vi "Initialize.vi"() -> ()   [LabVIEW 2010]
uses:
  <vilib>/Utility/miscctls.llb/LV3DPointTypeDef.ctl
  <vilib>/picture/3D Picture Control/NI_3D Picture Control.lvlib
  <vilib>/Analysis/NI_AALBase.lvlib
panel:
  in  "MagCal":bool caption="InitializeEEPROM"
  in  "Initialize EEPROM":bool caption="InitializeEEPROM"
  in  "ESCCal":bool caption="InitializeEEPROM"
  in  "TransmitterCal":bool caption="InitializeEEPROM"
  in  "AccelCal":bool caption="InitializeEEPROM"
  in  "GyroCal":bool caption="InitializeEEPROM"
  in  "Upload Flight Software":bool caption="InitializeEEPROM"
  out "Z Axis":cluster{dbl, dbl, dbl}(slide)={0.0, 519.4805194805194, -331.16883116883116} scale=-800.0..800.0
  out "Y Axis":cluster{dbl, dbl, dbl}(slide)={0.0, 519.4805194805194, -331.16883116883116} scale=-800.0..800.0
  out "X Axis":cluster{dbl, dbl, dbl}(slide)={0.0, 519.4805194805194, -331.16883116883116} scale=-800.0..800.0
  out "AUX3":dbl
  out "AUX2":dbl
  out "AUX1":dbl
  out "Mode":dbl
  out "Pitch":dbl
  out "Roll":dbl
  out "Yaw":dbl
  out "Throttle":dbl
  out "AUX3Bar":sgl(slide) scale=1000.0..2000.0
  out "AUX2Bar":sgl(slide) scale=1000.0..2000.0
  out "AUX1Bar":sgl(slide) scale=1000.0..2000.0
  out "ModeBar":sgl(slide) scale=1000.0..2000.0
  out "Right Stick":refnum<vi>(3d-picture)
  out "PitchBar":sgl(slide) scale=1000.0..2000.0
  out "RollBar":sgl(slide) scale=1000.0..2000.0
  out "Left Stick":refnum<vi>(3d-picture)
  out "ThrottleBar":sgl(slide) scale=1000.0..2000.0
  out "YawBar":sgl(slide) scale=1000.0..2000.0
  out "LargeInstructions":string
  out "AccelGUI":refnum<vi>(3d-picture)
  out "Instruction":string
  in  "OK":bool caption="InitializeEEPROM"
  in  "Cancel":bool caption="InitializeEEPROM"
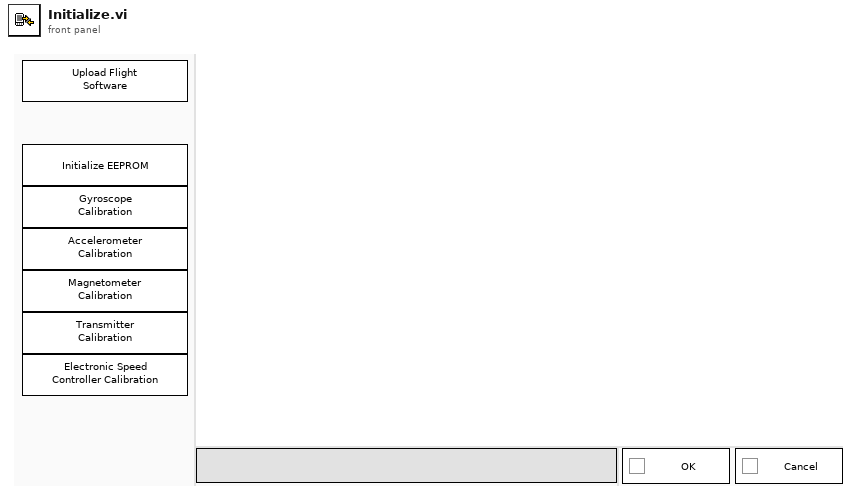
[diagram p1: front panel]
types:
  T1 = cluster{"Error":errorcluster, "GUIQueue":refnum<queue>, "TlmType":string, "Response":enum16{"Wait", "OK", "Cancel"}, "Data":dbl[][], "LeftStick":refnum<vi>, "RightStick":refnum<vi>, "XmitMax":dbl[], "XmitMin":dbl[], "NextState":string, "XmitCount":i32, "SubPanelData":string[][], "ModelRef":refnum<vi>, "Radians":dbl, "Z":sgl, "Y":sgl, "AccelIndex":i32, "AccelData":dbl[][], "AccelRaw":dbl[][], "AccelScaleFactor":dbl[], "AccelBias":dbl[], "MagMin":dbl[], "MagMax":dbl[], "IniData":string[][], "LeftStickScene":refnum<vi>, "RightStickScene":refnum<vi>, "WorkingFolder":path}
  T2 = enum8{"Enabled", "Disabled", "Disabled and Grayed Out"}
  T3 = typedef "LV3DPointTypeDef.ctl" = cluster{"X":sgl, "Y":sgl, "Z":sgl}
  T4 = cluster{"Red":sgl, "Green":sgl, "Blue":sgl, "Alpha":sgl}
  T5 = enum32{"invalid app kind", "Development System", "Run Time System", "Student Edition", "Embedded LabVIEW", "Evaluation", "Custom"}
  T6 = cluster{"State":string, "Reponse":enum16{"Wait", "OK", "Cancel"}}
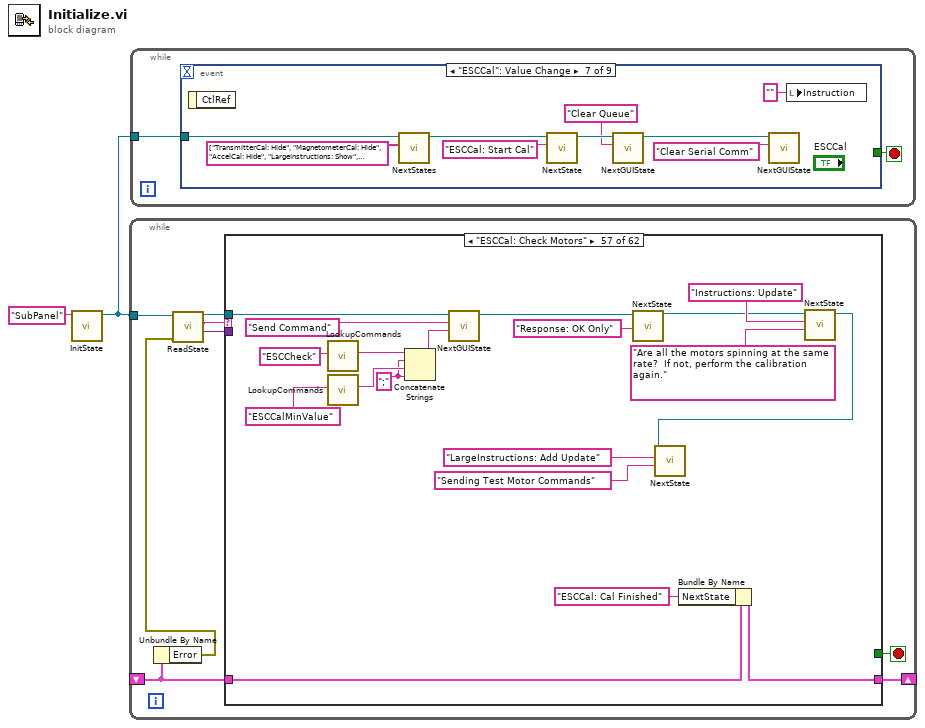
[diagram p0: block diagram]
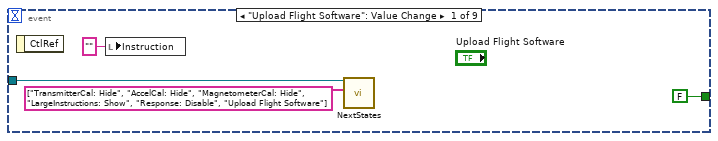
[diagram p2: hidden frame]
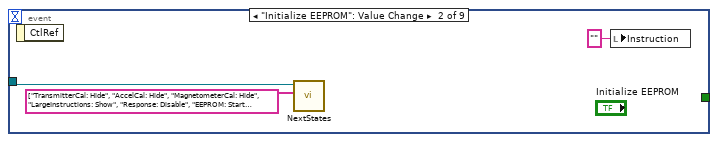
[diagram p3: hidden frame]
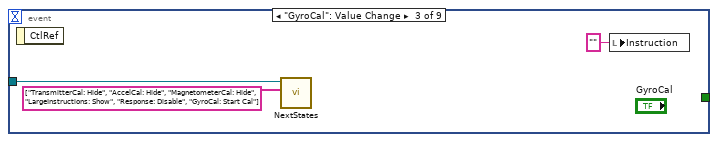
[diagram p4: hidden frame]
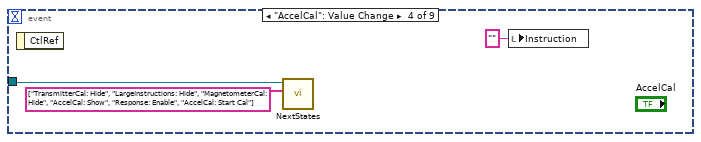
[diagram p5: hidden frame]
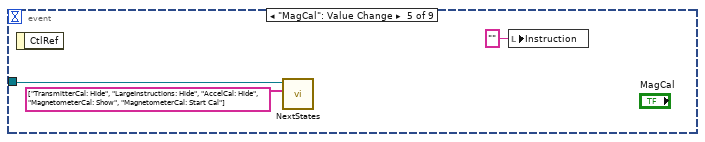
[diagram p6: hidden frame]
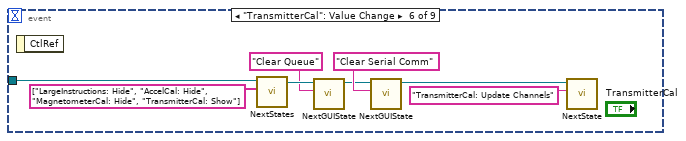
[diagram p7: hidden frame]
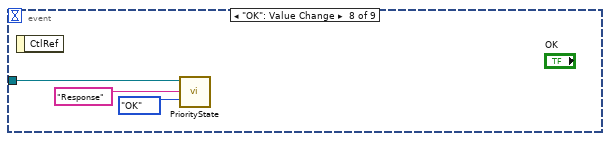
[diagram p8: hidden frame]
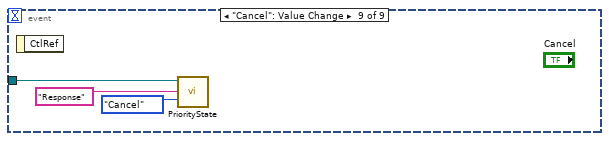
[diagram p9: hidden frame]
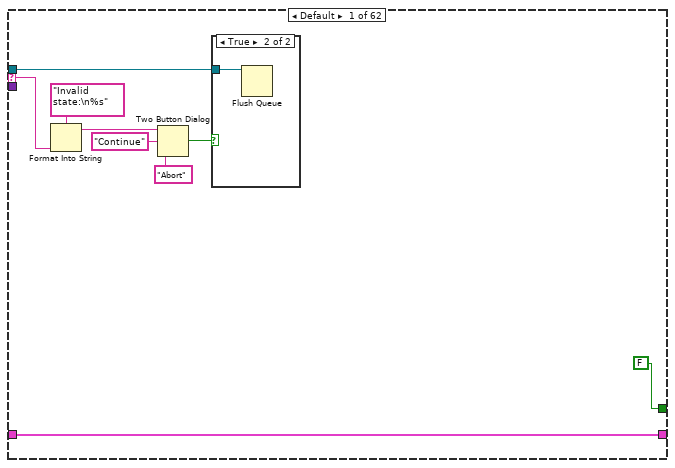
[diagram p10: hidden frame]
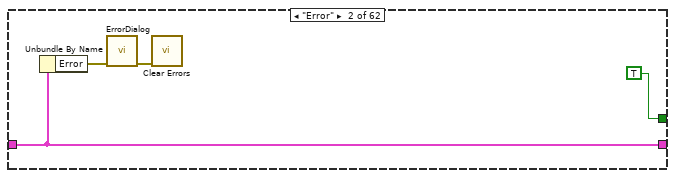
[diagram p12: hidden frame]
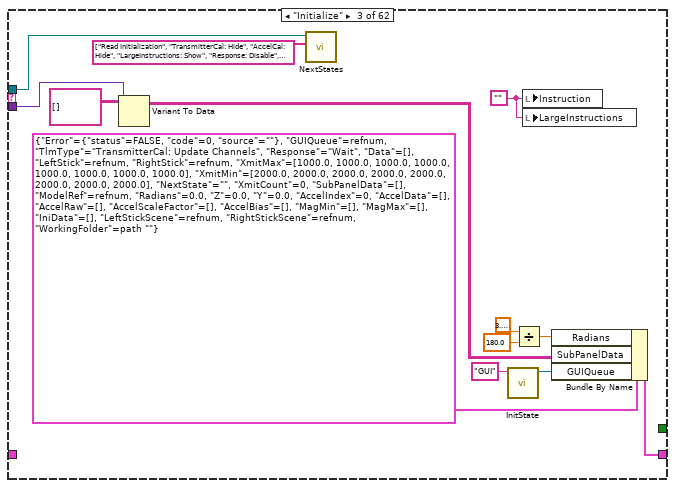
[diagram p13: hidden frame]
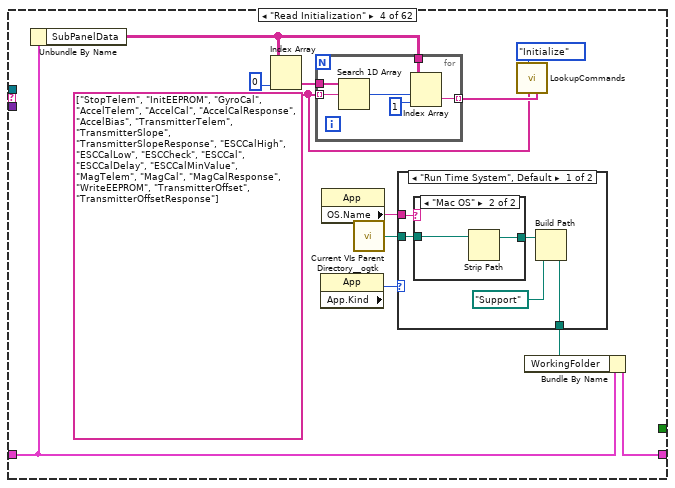
[diagram p14: hidden frame]
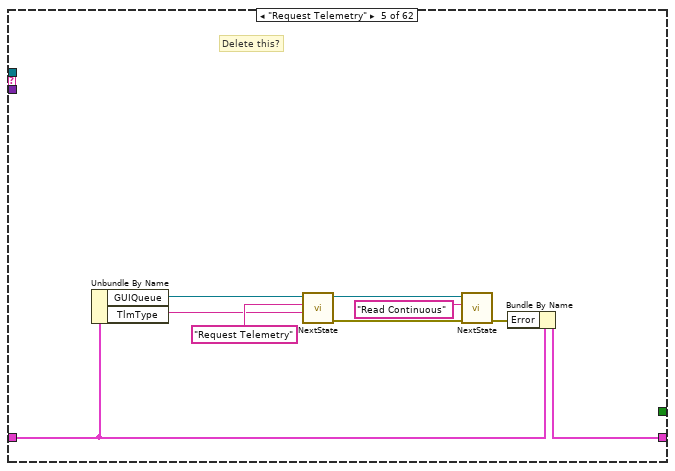
[diagram p17: hidden frame]
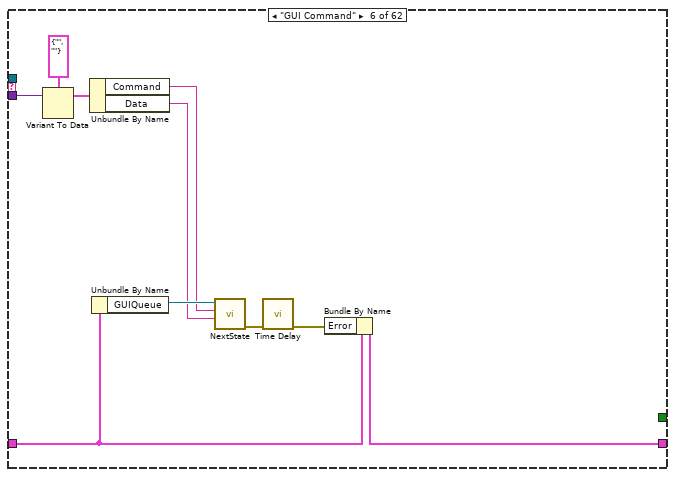
[diagram p18: hidden frame]
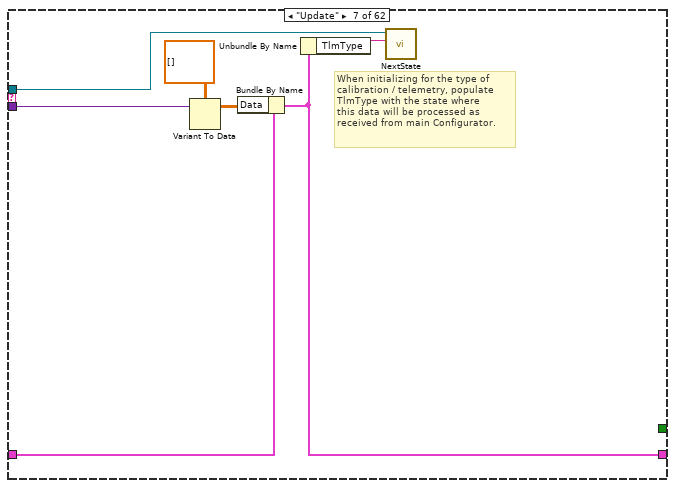
[diagram p19: hidden frame]
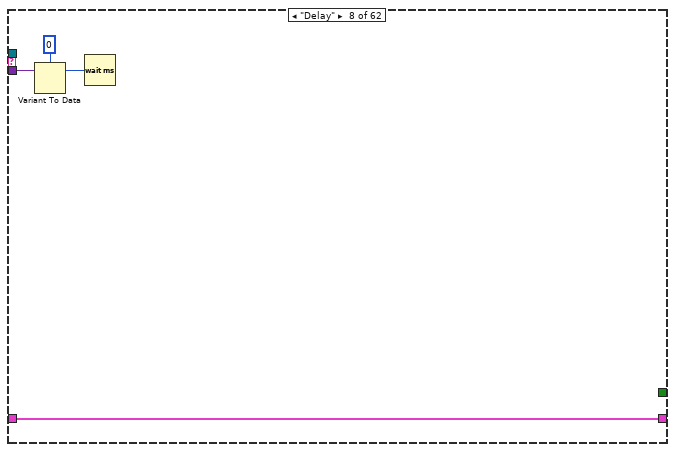
[diagram p20: hidden frame]
diagram:
  n1 = call "InitState.vi"("Name"="SubPanel" ("name (unnamed)")) -> ("Queue Out"=w1:refnum<queue>)  [unwired: 8 in, 1 out]
  n2 = while {
    tunnel: w1 -> [w7]
    shift-right: [w10] -> _
    shift-left: _ -> [w9]
    stop <- w8 stop-if-true
    n3 = Unbundle By Name(w9) -> ("Error"=w3:errorcluster)
    n4 = call "ReadState.vi"("Error In"=w3, "Queue In"=w7) -> ("Data"=w6:variant, "State"=w5:string, "Queue Out"=w4:refnum<queue>)  [unwired: 6 in, 1 out]
    n5 = case shown="\"ESCCal: Check Motors\"" w5 {
      tunnel: w4 -> [w11 _ w26 _ _ _ w86 _ w97 w104 w111 _ _ _ _ _ _ _ _ _ _ w171 w189 w217 _ w246 w266 _ w294 w323 w327 w356 w360 w389 w393 w422 w426 w458 w462 w491 _ w508 w560 w634 w650 w652 _ w695 w726 w756 w792 _ w886 w910 w944 w968 w983 w1002 _ w1030 _ w1085]
      selector: w5 -> [w17 _ _ _ _ _ _ _ _ _ _ _ _ _ _ _ _ _ _ _ w159 _ _ _ w232 _ _ _ _ _ _ _ _ _ _ _ _ _ _ _ _ _ _ _ _ _ w676 _ _ _ _ _ _ _ _ _ _ _ w1009 _ _ _]
      tunnel: w6 -> [_ _ w27 _ _ w74 w85 w94 _ _ w109 _ _ _ _ _ _ w144 w146 w155 _ _ _ _ _ _ w268 _ _ _ _ _ _ _ _ _ _ _ _ _ _ _ _ _ _ _ _ _ _ _ _ _ _ _ _ _ _ _ _ _ _ _]
      tunnel: [w16 w23 w36 w39 w70 w82 w88 w91 w95 w106 w110 w126 w130 w133 w135 w137 w138 w145 w149 w157 w162 w170 w200 w216 w233 w251 w265 w288 w304 w320 w334 w353 w367 w386 w400 w419 w433 w455 w469 w488 w495 w504 w554 w612 w648 w654 w677 w696 w719 w790 w826 w833 w882 w912 w948 w971 w989 w1006 w1008 w1021 w1041 w1082] -> w10
      tunnel: w9 -> [w16 w23 _ w40 w72 w83 w89 w91 w95 w106 w110 w126 w130 w133 w135 w137 w138 w145 w149 w157 w162 w170 w200 w216 w233 w252 w265 w288 w305 w321 w335 w354 w368 w387 w401 w420 w434 w456 w470 w489 w495 w505 w555 w613 w648 w655 w677 w697 w699 w774 w826 w834 w882 w913 w948 w971 w990 w1006 w1008 w1025 w1042 w1082]
      tunnel: [FALSE TRUE _ _ _ _ _ _ _ _ _ _ _ _ _ TRUE _ _ _ _ _ _ _ _ _ _ _ _ _ _ _ _ _ _ _ _ _ _ _ _ _ _ _ _ _ _ _ _ _ _ _ _ _ _ _ _ _ _ _ _ _ _] -> w8
      frame Default {
        n6 = Format Into String(format string="Invalid state:\n%s", w17) -> (resulting string=w18:string)  [unwired: 2 in, 1 out]
        n7 = Two Button Dialog(message=w18, 1:"Abort" ("F button name (\"Cancel\")"), 2:"Continue" ("T button name (\"OK\")")) -> (T button?=w12:bool)
        n8 = case shown="True" w12 {
          tunnel: w11 -> [_ w20]
          frame False {
          }
          frame True {
            n9 = Flush Queue(queue=w20) -> ()  [unwired: 1 in, 3 out]
          }
        }
      }
      frame "Error" {
        n10 = Unbundle By Name(w23) -> ("Error"=w22:errorcluster)
        n11 = call "ErrorDialog.vi"("error in"=w22) -> ("error out"=w21:errorcluster)  [unwired: 10 in]
        n12 = call <vilib>:"Clear Errors.vi"("error in (no error)"=w21) -> ()  [unwired: 6 in, 1 out]
      }
      frame "Initialize" {
        w32 = ""
        n13 = Variant To Data(Variant=w27, type=string[][] [] ("subarray")) -> (data=w25:string[][])  [unwired: 1 in, 1 out]
        n14 = call "NextStates.vi"("States"=string[] ["Read Initialization", "TransmitterCal: Hide", "AccelCal: Hide", "LargeInstructions: Show", "Response: Disable", "Show Welcome Message"], "Queue In"=w26) -> ()  [unwired: 8 in, 2 out]
        n15 = call "InitState.vi"("Name"="GUI") -> ("Queue Out"=w34:refnum<queue>)  [unwired: 8 in, 1 out]
        n16 = Divide(x=3.141592653589793, y=180.0) -> (x/y=w28:dbl)
        n17 = local write "Instruction"(w32) -> ()
        n18 = local write "LargeInstructions"(w32) -> ()
        n19 = Bundle By Name(cluster=T1 {"Error"={"status"=FALSE, "code"=0, "source"=""}, "GUIQueue"=refnum, "TlmType"="TransmitterCal: Update Channels", "Response"=enum."Wait", "Data"=[], "LeftStick"=refnum, "RightStick"=refnum, "XmitMax"=[1000.0, 1000.0, 1000.0, 1000.0, 1000.0, 1000.0, 1000.0, 1000.0], "XmitMin"=[2000.0, 2000.0, 2000.0, 2000.0, 2000.0, 2000.0, 2000.0, 2000.0], "NextState"="", "XmitCount"=0, "SubPanelData"=[], "ModelRef"=refnum, "Radians"=0.0, "Z"=0.0, "Y"=0.0, "AccelIndex"=0, "AccelData"=[], "AccelRaw"=[], "AccelScaleFactor"=[], "AccelBias"=[], "MagMin"=[], "MagMax"=[], "IniData"=[], "LeftStickScene"=refnum, "RightStickScene"=refnum, "WorkingFolder"=path ""}, "Radians"=w28, "SubPanelData"=w25, "GUIQueue"=w34) -> (w36:T1)
      }
      frame "Read Initialization" {
        w44 = string[] ["StopTelem", "InitEEPROM", "GyroCal", "AccelTelem", "AccelCal", "AccelCalResponse", "AccelBias", "TransmitterTelem", "TransmitterSlope", "TransmitterSlopeResponse", "ESCCalHigh", "ESCCalLow", "ESCCheck", "ESCCal", "ESCCalDelay", "ESCCalMinValue", "MagTelem", "MagCal", "MagCalResponse", "WriteEEPROM", "TransmitterOffset", "TransmitterOffsetResponse"]
        n20 = Unbundle By Name(w40) -> ("SubPanelData"=w47:string[][])
        n21 = Index Array(array=w47, index (col)=0 ("index (row)")) -> (element=w49:string[])  [unwired: 1 in]
        n22 = for {
          tunnel: w49 -> [w64]
          tunnel: w44 -> [w60] mode=indexing
          tunnel: w47 -> [w63]
          tunnel: [w59] -> w45 mode=indexing
          n23 = Search 1D Array(1D array=w64, element=w60) -> (index of element=w61:i32)  [unwired: 1 in]
          n24 = Index Array(array=w63, index (row)=w61, index (col)=1 ("disabled index (col)")) -> (element=w59:string)
        }
        n25 = property class="App"() -> ("App.Kind"=w43:T5)  [unwired: 2 in, 2 out]
        n26 = property class="App"() -> ("OS.Name"=w41:string)  [unwired: 2 in, 2 out]
        n27 = call <userlib>:"Current VIs Parent Directory__ogtk.vi"() -> ("Parent Directory (+ Relative)"=w42:path)  [unwired: 5 in]
        n28 = case shown="\"Run Time System\", Default" w43 {
          tunnel: [w54 w58] -> w38
          tunnel: w42 -> [w52 w58]
          tunnel: w41 -> [w50 _]
          frame "Run Time System", Default {
            n29 = case shown="\"Mac OS\"" w50 {
              tunnel: [w55 w57] -> w53
              tunnel: w52 -> [w55 w56]
              frame Default {
              }
              frame "Mac OS" {
                n30 = Strip Path(path=w56) -> (stripped path=w57:path)  [unwired: 1 out]
              }
            }
            n31 = Build Path(base path=w53, name or relative path=path "Support") -> (appended path=w54:path)
          }
          frame "Development System" {
          }
        }
        n32 = call "LookupCommands.vi"("CommandValues"=w45, "CommandNames"=w44, "Mode"=enum16{"Read", "Initialize"}."Initialize") -> ()  [unwired: 8 in, 1 out]
        n33 = Bundle By Name(cluster=w40, "WorkingFolder"=w38) -> (w39:T1)
      }
      frame "Request Telemetry" {
        # "Delete this?"
        n34 = Unbundle By Name(w72) -> ("GUIQueue"=w68:refnum<queue>, "TlmType"=w67:string)
        n35 = call "NextState.vi"("Data"=w67, "State"="Request Telemetry", "Queue In"=w68) -> ("Error Out"=w65:errorcluster, "Queue Out"=w66:refnum<queue>)  [unwired: 7 in]
        n36 = call "NextState.vi"("Error In"=w65, "State"="Read Continuous", "Queue In"=w66) -> ("Error Out"=w71:errorcluster)  [unwired: 7 in, 1 out]
        n37 = Bundle By Name(cluster=w72, "Error"=w71) -> (w70:T1)
      }
      frame "GUI Command" {
        n38 = Variant To Data(Variant=w74, type=cluster{"Command":string, "Data":string} {"Command"="", "Data"=""}) -> (data=w79:cluster{"Command":string, "Data":string})  [unwired: 1 in, 1 out]
        n39 = Unbundle By Name(w79) -> ("Command"=w76:string, "Data"=w75:string)
        n40 = Unbundle By Name(w83) -> ("GUIQueue"=w81:refnum<queue>)
        n41 = call "NextState.vi"("Data"=w75, "State"=w76, "Queue In"=w81) -> ("Error Out"=w78:errorcluster)  [unwired: 7 in, 1 out]
        n42 = call "Time Delay"("error in (no error)"=w78) -> ("error out"=w77:errorcluster)  [unwired: 10 in]
        n43 = Bundle By Name(cluster=w83, "Error"=w77) -> (w82:T1)
      }
      frame "Update" {
        # "When initializing for the type of\ncalibration / telemetry, populate\nTlmType with the state where\nthis data will be processed as\nreceived from main Configurator."
        n44 = Variant To Data(Variant=w85, type=dbl[][] []) -> (data=w84:dbl[][])  [unwired: 1 in, 1 out]
        n45 = Bundle By Name(cluster=w89, "Data"=w84) -> (w88:T1)
        n46 = Unbundle By Name(w88) -> ("TlmType"=w87:string)
        n47 = call "NextState.vi"("State"=w87, "Queue In"=w86) -> ()  [unwired: 8 in, 2 out]
      }
      frame "Delay" {
        n48 = Variant To Data(Variant=w94, type=u32 0 ("milliseconds to wait")) -> (data=w92:u32)  [unwired: 1 in, 1 out]
        n49 = Wait (ms)(milliseconds to wait=w92) -> ()  [unwired: 1 out]
      }
      frame "Wait For User" {
        n50 = Unbundle By Name(w95) -> ("Response"=w96:enum16{"Wait", "OK", "Cancel"})
        n51 = case shown="\"Wait\"" w96 {
          tunnel: w97 -> [_ w102]
          frame Default {
          }
          frame "Wait" {
            n52 = Bundle("State"="Wait For User", "Reponse"=enum16{"Wait", "OK", "Cancel"}."Wait") -> (w98:T6)  [unwired: 1 in]
            n53 = Enqueue Element At Opposite End(queue=w102, element=w98) -> ()  [unwired: 2 in, 3 out]
            n54 = Wait (ms)(milliseconds to wait=u32 100) -> ()  [unwired: 1 out]
          }
        }
      }
      frame "Show Welcome Message" {
        n55 = call "NextState.vi"("Data"="Welcome to the AeroQuad Configurator!\n\nThis tool is used to configure, calibrate and test your AeroQuad in preparation for flight.  Before using the Configurator, please install the Arduino IDE 1.0 or greater (found at www.arduino.cc) and install the proper drivers for your Arduino board to connect to your computer.\n\nTo setup your AeroQuad click on each of the buttons in the Initial Setup screen:\n - Upload Flight Software (advanced users can also upload directly from the Arduino IDE)\n - Initialize EEPROM (returns user configurable values to their default values)\n - Gyroscope Calibration\n - Accelerometer Calibration\n - Magnetometer Calibration (only valid with hardware configurations supporting this)\n - Transmitter Calibration\n - Electronic Speed Controller Calibration (perform this calibration with no propellers attached)\n\nAfter your AeroQuad has been properly setup, you can revisit the Initial Setup screen periodically to update  your AeroQuad configuration and calibrations as necessary.\n\nTo arm the AeroQuad motors, move the left transmitter stick to the lower right hand corner.  To disarm the motors, move the left transmitter stick to the lower left hand corner.  To perform a quick gyro/accel calibration move the left transmitter stick to the lower left hand corner and move the right transmitter stick to the lower right hand corner.\n\nFor additional help please visit www.AeroQuad.com to access our wiki documentation, help forums, and IRC chat.  Please practice safe flying, as multicopters can be dangerous if not flown with common sense.  Do as much testing as possible with the propellers not attached and only fly in approved R/C locations." ("State"), "State"="LargeInstructions: Update", "Queue In"=w104) -> ()  [unwired: 7 in, 2 out]
      }
      frame "Response" {
        w115 = enum16{"Wait", "OK", "Cancel"}."OK"  # Reponse
        # "To use the front panel OK and Cancel buttons:\nSet \"Next State\" to the state that needs to run right after the buttons are pressed.\nGo to the Reponse: Enable state to enable the buttons\nGo to Instructions: Update and send a message to tell user what happens when\n  buttons are pressed\nButtons wil automatically be disabled once either OK or Canel is pressed"
        n56 = Unbundle By Name(w110) -> ("NextState"=w112:string)
        n57 = Variant To Data(Variant=w109, type=w115) -> (data=w114:enum16{"Wait", "OK", "Cancel"})  [unwired: 1 in, 1 out]
        n58 = Equal?(x=w114, y=w115) -> (x = y?=w113:bool)
        n59 = case shown="True" w113 {
          tunnel: w112 -> [_ w121]
          tunnel: w111 -> [w119 w122]
          tunnel: [w116 w120] -> w108
          frame False {
            n60 = call "NextState.vi"("Data"="Operation cancelled." ("State"), "State"="Instructions: Update", "Queue In"=w119) -> ("Queue Out"=w116:refnum<queue>)  [unwired: 7 in, 1 out]
          }
          frame True {
            n61 = call "NextState.vi"("State"=w121, "Queue In"=w122) -> ("Queue Out"=w120:refnum<queue>)  [unwired: 8 in, 1 out]
          }
        }
        n62 = call "NextState.vi"("State"="Response: Disable", "Queue In"=w108) -> ()  [unwired: 8 in, 2 out]
      }
      frame "Response: Enable" {
        n63 = local write "Instruction"("" ("Instruction")) -> ()
        n64 = property on="Cancel" class="Bool"("DisabledEnum"=T2."Enabled" ("Disabled")) -> ()  [unwired: 2 in, 2 out]
        n65 = property on="OK" class="Bool"("DisabledEnum"=T2."Enabled" ("Disabled")) -> ()  [unwired: 2 in, 2 out]
      }
      frame "Response: OK Only" {
        n66 = local write "Instruction"("" ("Instruction")) -> ()
        n67 = property on="Cancel" class="Bool"("DisabledEnum"=T2."Disabled and Grayed Out" ("Disabled")) -> ()  [unwired: 2 in, 2 out]
        n68 = property on="OK" class="Bool"("DisabledEnum"=T2."Enabled" ("Disabled")) -> ()  [unwired: 2 in, 2 out]
      }
      frame "Response: Disable" {
        n69 = property on="Cancel" class="Bool"("DisabledEnum"=T2."Disabled and Grayed Out" ("Disabled")) -> ()  [unwired: 2 in, 2 out]
        n70 = property on="OK" class="Bool"("DisabledEnum"=T2."Disabled and Grayed Out" ("Disabled")) -> ()  [unwired: 2 in, 2 out]
      }
      frame "Temporary" {
        n71 = One Button Dialog(message="This feature under contruction.") -> ()  [unwired: 1 in, 1 out]
      }
      frame "Shutdown" {
      }
      frame "----------" {
      }
      frame "Instructions: Update" {
        w141 = "" ("Instruction")
        n72 = Variant To Data(Variant=w144, type=w141) -> (data=w139:string)  [unwired: 1 in, 1 out]
        n73 = Equal?(x=w139, y="Calibration... 0 %") -> (x = y?=w142:bool)
        n74 = Select(t=w141, s=w142, f=w139) -> (s? t:f=→"Instruction":string)
      }
      frame "LargeInstructions: Update" {
        n75 = Variant To Data(Variant=w146, type="" ("Instruction")) -> (data=→"LargeInstructions":string)  [unwired: 1 in, 1 out]
      }
      frame "LargeInstructions: Add Update" {
        n76 = Variant To Data(Variant=w155, type="" ("Instruction")) -> (data=w154:string)  [unwired: 1 in, 1 out]
        n77 = local read "LargeInstructions"() -> (w153:string)
        n78 = Concatenate Strings(w153, "\n\n**********\n\n" ("string"), w154) -> (w151:string)
        n79 = property on="LargeInstructions" class="Str"("Value"=w151, "Text.Scroll Position"=u32 1024) -> ()  [unwired: 2 in, 2 out]
      }
      frame "LargeInstructions: Hide", "LargeInstructions: Show" {
        n80 = Match Pattern(string=w159, regular expression="Show") -> (offset past match=w161:i32)  [unwired: 1 in, 3 out]
        n81 = Greater Or Equal To 0?(x=w161) -> (x >= 0?=w158:bool)
        n82 = property on="LargeInstructions" class="Str"("Visible"=w158) -> ()  [unwired: 2 in, 2 out]
      }
      frame "Upload Flight Software" {
        n83 = call "NextGUIState.vi"("GUI State"="Disconnect" ("State"), "Queue In"=w171) -> ("Queue Out"=w166:refnum<queue>)  [unwired: 8 in, 1 out]
        n84 = flat-sequence {
          tunnel: w166 -> [w176]
          tunnel: [w176] -> w169
          tunnel: [w175] -> w168
          tunnel: [w177] -> w164
          tunnel: [w182] -> w165
          tunnel: w169 -> [w182]
          tunnel: w168 -> [w177]
          tunnel: [w178] -> w163
          frame #0 {
            n85 = call "AeroQuadUploader.vi"() -> ("Com Port Out"=w175:refnum<visa-resource-name>)  [unwired: 11 in]
          }
          frame #1 {
            n86 = call "TestUsbSerialPort.vi"("Serial Port To Test"=w177) -> ()  [unwired: 9 in, 2 out]
            n87 = Two Button Dialog(message="Would you like to auto-connect to the AeroQuad?", 1:"No", 2:"Yes") -> (T button?=w178:bool)
          }
        }
        n88 = case shown="True" w163 {
          tunnel: w165 -> [_ w174]
          tunnel: w164 -> [_ w172]
          frame False {
          }
          frame True {
            n89 = call "NextGUIState.vi"("State Argument"=w172, "GUI State"="Remote Open Port" ("State Argument"), "Queue In"=w174) -> ()  [unwired: 7 in, 2 out]
          }
        }
      }
      frame "EEPROM: Start Initialization" {
        n90 = call "NextGUIState.vi"("GUI State"="Lock User Controls" ("State"), "Queue In"=w189) -> ("Queue Out"=w190:refnum<queue>)  [unwired: 8 in, 1 out]
        n91 = call "NextGUIState.vi"("State Argument"="Please wait, updating EEPROM..." ("State"), "GUI State"="Status" ("State"), "Queue In"=w190) -> ("Queue Out"=w211:refnum<queue>)  [unwired: 7 in, 1 out]
        n92 = call "NextGUIState.vi"("GUI State"="Clear Queue", "Queue In"=w211) -> ("Queue Out"=w208:refnum<queue>)  [unwired: 8 in, 1 out]
        n93 = call "LookupCommands.vi"("CommandName"="InitEEPROM") -> ("CommandValue"=w198:string)  [unwired: 10 in]
        n94 = call "NextGUIState.vi"("GUI State"="Clear Serial Comm", "Queue In"=w208) -> ("Queue Out"=w206:refnum<queue>)  [unwired: 8 in, 1 out]
        n95 = call "NextGUIState.vi"("State Argument"=w198, "GUI State"="Send Command" ("State"), "Queue In"=w206) -> ("Queue Out"=w212:refnum<queue>)  [unwired: 7 in, 1 out]
        n96 = call "NextGUIState.vi"("State Argument"="1000", "GUI State"="Delay String", "Queue In"=w212) -> ("Queue Out"=w193:refnum<queue>)  [unwired: 7 in, 1 out]
        n97 = call "NextGUIState.vi"("GUI State"="Update Parameters" ("State"), "Queue In"=w193) -> ("Queue Out"=w187:refnum<queue>)  [unwired: 8 in, 1 out]
        n98 = call "LookupCommands.vi"("CommandName"="WriteEEPROM") -> ("CommandValue"=w196:string)  [unwired: 10 in]
        n99 = call "NextGUIState.vi"("State Argument"=w196, "GUI State"="Send Command" ("State"), "Queue In"=w187) -> ("Queue Out"=w186:refnum<queue>)  [unwired: 7 in, 1 out]
        n100 = call "NextGUIState.vi"("State Argument"="1000", "GUI State"="Delay String", "Queue In"=w186) -> ("Queue Out"=w185:refnum<queue>)  [unwired: 7 in, 1 out]
        n101 = call "NextGUIState.vi"("State Argument"="EEPROM Initialized" ("State"), "GUI State"="Status" ("State"), "Queue In"=w185) -> ("Queue Out"=w183:refnum<queue>)  [unwired: 7 in, 1 out]
        n102 = call "NextGUIState.vi"("GUI State"="Unlock User Controls" ("State"), "Queue In"=w183) -> ()  [unwired: 8 in, 2 out]
      }
      frame "GyroCal: Start Cal" {
        n103 = call "NextGUIState.vi"("GUI State"="Clear Queue", "Queue In"=w217) -> ("Queue Out"=w227:refnum<queue>)  [unwired: 8 in, 1 out]
        n104 = call "NextGUIState.vi"("GUI State"="Clear Serial Comm", "Queue In"=w227) -> ("Queue Out"=w224:refnum<queue>)  [unwired: 8 in, 1 out]
        n105 = call "LookupCommands.vi"("CommandName"="GyroCal") -> ("CommandValue"=w214:string)  [unwired: 10 in]
        n106 = call "NextGUIState.vi"("State Argument"="Starting Gyroscope Calibration" ("State"), "GUI State"="Status" ("State"), "Queue In"=w224) -> ("Queue Out"=w225:refnum<queue>)  [unwired: 7 in, 1 out]
        n107 = call "NextGUIState.vi"("State Argument"=w214, "GUI State"="Send Command", "Queue In"=w225) -> ("Queue Out"=w218:refnum<queue>)  [unwired: 7 in, 1 out]
        n108 = call "NextGUIState.vi"("State Argument"="Gyroscope calibration complete" ("State"), "GUI State"="Status" ("State"), "Queue In"=w218) -> ()  [unwired: 7 in, 2 out]
      }
      frame "AccelCal: Hide", "AccelCal: Show" {
        n109 = Match Pattern(string=w232, regular expression="Show") -> (offset past match=w230:i32)  [unwired: 1 in, 3 out]
        n110 = Greater Or Equal To 0?(x=w230) -> (x >= 0?=w229:bool)
        n111 = property on="AccelGUI" class="SceneGraphDisp (strict)"("Visible"=w229) -> ()  [unwired: 2 in, 2 out]
      }
      frame "AccelCal: Start Cal" {
        w238 = dbl[][] [] ("AccelData")
        n112 = Unbundle By Name(w252) -> ("WorkingFolder"=w237:path, "SubPanelData"=w254:string[][])
        n113 = Index Array(array=w254, index (col)=0 ("index (row)")) -> (element=w255:string[])  [unwired: 1 in]
        n114 = Search 1D Array(1D array=w255, element="Filename") -> (index of element=w258:i32)  [unwired: 1 in]
        n115 = call "NextState.vi"("State"="AccelCal: Update Camera", "Queue In"=w246) -> ("Queue Out"=w247:refnum<queue>)  [unwired: 8 in, 1 out]
        n116 = Index Array(array=w254, index (row)=w258, index (col)=1 ("index (row)")) -> (element=w250:string)
        n117 = Build Path(base path=w237, name or relative path=w250) -> (appended path=w241:path)
        n118 = call <vilib>:"Create Object.vi"() -> ("Scene:New Object"=w262:refnum<vi>)  [unwired: 2 in, 9 out]
        n119 = call <vilib>:"Load STL Geometry.vi"("Model File"=w241) -> ("error out"=w261:errorcluster, "New Mesh Refnum"=w263:refnum<vi>)  [unwired: 9 in]
        n120 = invoke class="SceneObject" method="Set Drawable"(reference=w262, error in=w261, "Drawable"=w263) -> (reference out=w259:refnum<vi>, error out=w260:errorcluster)  [unwired: 1 in, 2 out]
        n121 = call "NextState.vi"("State"="AccelCal: Display Right Side Up", "Queue In"=w247) -> ("Queue Out"=w239:refnum<queue>)  [unwired: 8 in, 1 out]
        n122 = Bundle By Name(cluster=w252, "AccelIndex"=0, "AccelData"=w238, "AccelRaw"=w238, "Y"=sgl -38.0, "Z"=sgl 15.0, "TlmType"="AccelCal: Update", "ModelRef"=w259, "Error"=w260) -> (w251:T1)
        n123 = call "NextState.vi"("State"="AccelCal: Update Display", "Queue In"=w239) -> ("Queue Out"=w234:refnum<queue>)  [unwired: 8 in, 1 out]
        n124 = call "NextGUIState.vi"("State Argument"="Performing Accelerometer Calibration" ("State"), "GUI State"="Status" ("State"), "Queue In"=w234) -> ()  [unwired: 7 in, 2 out]
      }
      frame "AccelCal: Request Telemetry" {
        # "This will automatically go\nto AccelCal: Update\nto store data"
        n125 = Variant To Data(Variant=w268, type=FALSE) -> (data=w264:bool)  [unwired: 1 in, 1 out]
        n126 = case shown="True" w264 {
          tunnel: w266 -> [w274 w285]
          frame False {
            n127 = call "NextGUIState.vi"("GUI State"="Clear Queue" ("State"), "Queue In"=w274) -> ("Queue Out"=w276:refnum<queue>)  [unwired: 8 in, 1 out]
            n128 = call "NextGUIState.vi"("GUI State"="Clear Serial Comm" ("State"), "Queue In"=w276) -> ("Queue Out"=w272:refnum<queue>)  [unwired: 8 in, 1 out]
            n129 = local write "Instruction"("" ("Instruction")) -> ()
            n130 = call "LookupCommands.vi"("CommandName"="StopTelem") -> ("CommandValue"=w269:string)  [unwired: 10 in]
            n131 = call "NextGUIState.vi"("State Argument"=w269, "GUI State"="Request Telemetry" ("State"), "Queue In"=w272) -> ()  [unwired: 7 in, 2 out]
          }
          frame True {
            n132 = call "LookupCommands.vi"("CommandName"="AccelTelem") -> ("CommandValue"=w278:string)  [unwired: 10 in]
            n133 = call "NextGUIState.vi"("State Argument"=w278, "GUI State"="Request Telemetry" ("State"), "Queue In"=w285) -> ("Queue Out"=w283:refnum<queue>)  [unwired: 7 in, 1 out]
            n134 = call "NextGUIState.vi"("GUI State"="Read Continuous", "Queue In"=w283) -> ("Queue Out"=w280:refnum<queue>)  [unwired: 8 in, 1 out]
            n135 = call "NextState.vi"("State"="Response: Disable", "Queue In"=w280) -> ()  [unwired: 8 in, 2 out]
          }
        }
      }
      frame "AccelCal: Update Camera" {
        w290 = T3 {"X"=0.0, "Y"=0.0, "Z"=0.0} ("Target")
        n136 = Unbundle By Name(w288) -> ("Y"=w287:sgl, "Z"=w286:sgl)
        n137 = Bundle By Name(cluster=w290, "Y"=w287, "Z"=w286) -> (w289:T3)
        n138 = invoke on="AccelGUI" class="SceneGraphDisp (strict)" method="Setup Camera"("Camera Position"=w289, "Target"=w290, "Up Direction"=T3 {"X"=0.0, "Y"=1.0, "Z"=1.0} ("Target")) -> ()  [unwired: 3 in, 6 out]
      }
      frame "AccelCal: Display Right Side Up" {
        n139 = Unbundle By Name(w305) -> ("Radians"=w311:dbl, "ModelRef"=w317:refnum<vi>)
        n140 = call <vilib>:"Clear Transformation.vi"("Object Refnum In"=w317) -> ("Object Refnum Out"=w310:refnum<vi>)  [unwired: 9 in, 1 out]
        n141 = Compound Arithmetic op=MULTIPLY(0.0 ("value"), w311) -> (w313:dbl)
        n142 = call "NextState.vi"("State"="AccelCal: Update Camera", "Queue In"=w294) -> ("Queue Out"=w293:refnum<queue>)  [unwired: 8 in, 1 out]
        n143 = call <vilib>:"Rotate Object.vi"("Angle"=w313, "Axis"=cluster{"X":sgl, "Y":sgl, "Z":sgl} {"X"=0.0, "Y"=1.0, "Z"=0.0}, "Scene.Object In"=w310) -> ("Scene.Object Out"=w314:refnum<vi>)  [unwired: 7 in, 1 out]
        n144 = Compound Arithmetic op=MULTIPLY(0.0 ("value"), w311) -> (w312:dbl)
        n145 = call <vilib>:"Rotate Object.vi"("Angle"=w312, "Axis"=cluster{"X":sgl, "Y":sgl, "Z":sgl} {"X"=1.0, "Y"=0.0, "Z"=0.0}, "Scene.Object In"=w314) -> ("Scene.Object Out"=w309:refnum<vi>)  [unwired: 7 in, 1 out]
        n146 = Compound Arithmetic op=MULTIPLY(0.0 ("value"), w311) -> (w307:dbl)
        n147 = call <vilib>:"Rotate Object.vi"("Angle"=w307, "Axis"=cluster{"X":sgl, "Y":sgl, "Z":sgl} {"X"=0.0, "Y"=0.0, "Z"=1.0}, "Scene.Object In"=w309) -> ("Scene.Object Out"=w306:refnum<vi>)  [unwired: 7 in, 1 out]
        n148 = call "NextState.vi"("State"="Response: Enable", "Queue In"=w293) -> ("Queue Out"=w295:refnum<queue>)  [unwired: 8 in, 1 out]
        n149 = Bundle By Name(cluster=w305, "Z"=sgl 0.0, "NextState"="AccelCal: Wait Right Side Up", "ModelRef"=w306) -> (w304:T1)
        n150 = call "NextState.vi"("Data"="Place the AeroQuad motionless on a flat surface." ("State"), "State"="Instructions: Update", "Queue In"=w295) -> ()  [unwired: 7 in, 2 out]
      }
      frame "AccelCal: Wait Right Side Up" {
        n151 = call "NextState.vi"("Data"=TRUE, "State"="AccelCal: Request Telemetry", "Queue In"=w323) -> ()  [unwired: 7 in, 2 out]
        n152 = Bundle By Name(cluster=w321, "AccelRaw"=dbl[][] [] ("AccelData"), "AccelIndex"=0, "NextState"="AccelCal: Display Upside Down") -> (w320:T1)
      }
      frame "AccelCal: Display Upside Down" {
        n153 = Unbundle By Name(w335) -> ("Radians"=w344:dbl, "ModelRef"=w350:refnum<vi>)
        n154 = call <vilib>:"Clear Transformation.vi"("Object Refnum In"=w350) -> ("Object Refnum Out"=w343:refnum<vi>)  [unwired: 9 in, 1 out]
        n155 = call "NextState.vi"("State"="Response: Enable", "Queue In"=w327) -> ("Queue Out"=w329:refnum<queue>)  [unwired: 8 in, 1 out]
        n156 = Compound Arithmetic op=MULTIPLY(180.0 ("value"), w344) -> (w346:dbl)
        n157 = call <vilib>:"Rotate Object.vi"("Angle"=w346, "Axis"=cluster{"X":sgl, "Y":sgl, "Z":sgl} {"X"=0.0, "Y"=1.0, "Z"=0.0}, "Scene.Object In"=w343) -> ("Scene.Object Out"=w347:refnum<vi>)  [unwired: 7 in, 1 out]
        n158 = Compound Arithmetic op=MULTIPLY(0.0 ("value"), w344) -> (w345:dbl)
        n159 = call <vilib>:"Rotate Object.vi"("Angle"=w345, "Axis"=cluster{"X":sgl, "Y":sgl, "Z":sgl} {"X"=1.0, "Y"=0.0, "Z"=0.0}, "Scene.Object In"=w347) -> ("Scene.Object Out"=w342:refnum<vi>)  [unwired: 7 in, 1 out]
        n160 = Compound Arithmetic op=MULTIPLY(0.0 ("value"), w344) -> (w340:dbl)
        n161 = call "NextState.vi"("Data"="Place the AeroQuad upside down." ("State"), "State"="Instructions: Update", "Queue In"=w329) -> ("Queue Out"=w326:refnum<queue>)  [unwired: 7 in, 1 out]
        n162 = call <vilib>:"Rotate Object.vi"("Angle"=w340, "Axis"=cluster{"X":sgl, "Y":sgl, "Z":sgl} {"X"=0.0, "Y"=0.0, "Z"=1.0}, "Scene.Object In"=w342) -> ("Scene.Object Out"=w339:refnum<vi>)  [unwired: 7 in, 1 out]
        n163 = Bundle By Name(cluster=w335, "NextState"="AccelCal: Wait Upside Side Down", "ModelRef"=w339) -> (w334:T1)
        n164 = call "NextState.vi"("State"="AccelCal: Update Display", "Queue In"=w326) -> ()  [unwired: 8 in, 2 out]
      }
      frame "AccelCal: Wait Upside Side Down" {
        n165 = call "NextState.vi"("Data"=TRUE, "State"="AccelCal: Request Telemetry", "Queue In"=w356) -> ()  [unwired: 7 in, 2 out]
        n166 = Bundle By Name(cluster=w354, "AccelRaw"=dbl[][] [] ("AccelData"), "AccelIndex"=0, "NextState"="AccelCal: Display Left Edge Down") -> (w353:T1)
      }
      frame "AccelCal: Display Left Edge Down" {
        n167 = Unbundle By Name(w368) -> ("Radians"=w377:dbl, "ModelRef"=w383:refnum<vi>)
        n168 = call <vilib>:"Clear Transformation.vi"("Object Refnum In"=w383) -> ("Object Refnum Out"=w376:refnum<vi>)  [unwired: 9 in, 1 out]
        n169 = Compound Arithmetic op=MULTIPLY(-90.0 ("value"), w377) -> (w379:dbl)
        n170 = call "NextState.vi"("State"="AccelCal: Update Display", "Queue In"=w360) -> ("Queue Out"=w359:refnum<queue>)  [unwired: 8 in, 1 out]
        n171 = call <vilib>:"Rotate Object.vi"("Angle"=w379, "Axis"=cluster{"X":sgl, "Y":sgl, "Z":sgl} {"X"=0.0, "Y"=1.0, "Z"=0.0}, "Scene.Object In"=w376) -> ("Scene.Object Out"=w380:refnum<vi>)  [unwired: 7 in, 1 out]
        n172 = Compound Arithmetic op=MULTIPLY(0.0 ("value"), w377) -> (w378:dbl)
        n173 = call <vilib>:"Rotate Object.vi"("Angle"=w378, "Axis"=cluster{"X":sgl, "Y":sgl, "Z":sgl} {"X"=1.0, "Y"=0.0, "Z"=0.0}, "Scene.Object In"=w380) -> ("Scene.Object Out"=w375:refnum<vi>)  [unwired: 7 in, 1 out]
        n174 = Compound Arithmetic op=MULTIPLY(0.0 ("value"), w377) -> (w373:dbl)
        n175 = call "NextState.vi"("State"="Response: Enable", "Queue In"=w359) -> ("Queue Out"=w362:refnum<queue>)  [unwired: 8 in, 1 out]
        n176 = call <vilib>:"Rotate Object.vi"("Angle"=w373, "Axis"=cluster{"X":sgl, "Y":sgl, "Z":sgl} {"X"=0.0, "Y"=0.0, "Z"=1.0}, "Scene.Object In"=w375) -> ("Scene.Object Out"=w372:refnum<vi>)  [unwired: 7 in, 1 out]
        n177 = Bundle By Name(cluster=w368, "NextState"="AccelCal: Wait Left Edge Down", "ModelRef"=w372) -> (w367:T1)
        n178 = call "NextState.vi"("Data"="Place the AeroQuad left edge down." ("State"), "State"="Instructions: Update", "Queue In"=w362) -> ()  [unwired: 7 in, 2 out]
      }
      frame "AccelCal: Wait Left Edge Down" {
        n179 = call "NextState.vi"("Data"=TRUE, "State"="AccelCal: Request Telemetry", "Queue In"=w389) -> ()  [unwired: 7 in, 2 out]
        n180 = Bundle By Name(cluster=w387, "AccelRaw"=dbl[][] [] ("AccelData"), "AccelIndex"=0, "NextState"="AccelCal: Display Right Edge Down") -> (w386:T1)
      }
      frame "AccelCal: Display Right Edge Down" {
        n181 = Unbundle By Name(w401) -> ("Radians"=w410:dbl, "ModelRef"=w416:refnum<vi>)
        n182 = call <vilib>:"Clear Transformation.vi"("Object Refnum In"=w416) -> ("Object Refnum Out"=w409:refnum<vi>)  [unwired: 9 in, 1 out]
        n183 = Compound Arithmetic op=MULTIPLY(90.0 ("value"), w410) -> (w412:dbl)
        n184 = call "NextState.vi"("State"="AccelCal: Update Display", "Queue In"=w393) -> ("Queue Out"=w392:refnum<queue>)  [unwired: 8 in, 1 out]
        n185 = call <vilib>:"Rotate Object.vi"("Angle"=w412, "Axis"=cluster{"X":sgl, "Y":sgl, "Z":sgl} {"X"=0.0, "Y"=1.0, "Z"=0.0}, "Scene.Object In"=w409) -> ("Scene.Object Out"=w413:refnum<vi>)  [unwired: 7 in, 1 out]
        n186 = Compound Arithmetic op=MULTIPLY(0.0 ("value"), w410) -> (w411:dbl)
        n187 = call <vilib>:"Rotate Object.vi"("Angle"=w411, "Axis"=cluster{"X":sgl, "Y":sgl, "Z":sgl} {"X"=1.0, "Y"=0.0, "Z"=0.0}, "Scene.Object In"=w413) -> ("Scene.Object Out"=w408:refnum<vi>)  [unwired: 7 in, 1 out]
        n188 = Compound Arithmetic op=MULTIPLY(0.0 ("value"), w410) -> (w406:dbl)
        n189 = call "NextState.vi"("State"="Response: Enable", "Queue In"=w392) -> ("Queue Out"=w395:refnum<queue>)  [unwired: 8 in, 1 out]
        n190 = call <vilib>:"Rotate Object.vi"("Angle"=w406, "Axis"=cluster{"X":sgl, "Y":sgl, "Z":sgl} {"X"=0.0, "Y"=0.0, "Z"=1.0}, "Scene.Object In"=w408) -> ("Scene.Object Out"=w405:refnum<vi>)  [unwired: 7 in, 1 out]
        n191 = Bundle By Name(cluster=w401, "NextState"="AccelCal: Wait Right Edge Down", "ModelRef"=w405) -> (w400:T1)
        n192 = call "NextState.vi"("Data"="Place the AeroQuad right edge down." ("State"), "State"="Instructions: Update", "Queue In"=w395) -> ()  [unwired: 7 in, 2 out]
      }
      frame "AccelCal: Wait Right Edge Down" {
        n193 = call "NextState.vi"("Data"=TRUE, "State"="AccelCal: Request Telemetry", "Queue In"=w422) -> ()  [unwired: 7 in, 2 out]
        n194 = Bundle By Name(cluster=w420, "AccelRaw"=dbl[][] [] ("AccelData"), "AccelIndex"=0, "NextState"="AccelCal: Display Rear Edge Down") -> (w419:T1)
      }
      frame "AccelCal: Display Rear Edge Down" {
        n195 = Unbundle By Name(w434) -> ("Radians"=w443:dbl, "ModelRef"=w449:refnum<vi>)
        n196 = call <vilib>:"Clear Transformation.vi"("Object Refnum In"=w449) -> ("Object Refnum Out"=w442:refnum<vi>)  [unwired: 9 in, 1 out]
        n197 = Compound Arithmetic op=MULTIPLY(0.0 ("value"), w443) -> (w445:dbl)
        n198 = call "NextState.vi"("State"="AccelCal: Update Display", "Queue In"=w426) -> ("Queue Out"=w425:refnum<queue>)  [unwired: 8 in, 1 out]
        n199 = call <vilib>:"Rotate Object.vi"("Angle"=w445, "Axis"=cluster{"X":sgl, "Y":sgl, "Z":sgl} {"X"=0.0, "Y"=1.0, "Z"=0.0}, "Scene.Object In"=w442) -> ("Scene.Object Out"=w446:refnum<vi>)  [unwired: 7 in, 1 out]
        n200 = Compound Arithmetic op=MULTIPLY(90.0 ("value"), w443) -> (w444:dbl)
        n201 = call <vilib>:"Rotate Object.vi"("Angle"=w444, "Axis"=cluster{"X":sgl, "Y":sgl, "Z":sgl} {"X"=1.0, "Y"=0.0, "Z"=0.0}, "Scene.Object In"=w446) -> ("Scene.Object Out"=w441:refnum<vi>)  [unwired: 7 in, 1 out]
        n202 = Compound Arithmetic op=MULTIPLY(0.0 ("value"), w443) -> (w439:dbl)
        n203 = call <vilib>:"Rotate Object.vi"("Angle"=w439, "Axis"=cluster{"X":sgl, "Y":sgl, "Z":sgl} {"X"=0.0, "Y"=0.0, "Z"=1.0}, "Scene.Object In"=w441) -> ("Scene.Object Out"=w438:refnum<vi>)  [unwired: 7 in, 1 out]
        n204 = call "NextState.vi"("State"="Response: Enable", "Queue In"=w425) -> ("Queue Out"=w428:refnum<queue>)  [unwired: 8 in, 1 out]
        n205 = Bundle By Name(cluster=w434, "NextState"="AccelCal: Wait Rear Edge Down", "ModelRef"=w438) -> (w433:T1)
        n206 = call "NextState.vi"("Data"="Place the AeroQuad rear edge down.  The arrow indicates the front of the AeroQuad." ("State"), "State"="Instructions: Update", "Queue In"=w428) -> ()  [unwired: 7 in, 2 out]
      }
      frame "AccelCal: Wait Rear Edge Down" {
        n207 = call "NextState.vi"("Data"=TRUE, "State"="AccelCal: Request Telemetry", "Queue In"=w458) -> ("Queue Out"=w452:refnum<queue>)  [unwired: 7 in, 1 out]
        n208 = call "NextState.vi"("Data"="Calibrating..." ("State"), "State"="Instructions: Update", "Queue In"=w452) -> ()  [unwired: 7 in, 2 out]
        n209 = Bundle By Name(cluster=w456, "AccelRaw"=dbl[][] [] ("AccelData"), "AccelIndex"=0, "NextState"="AccelCal: Display Front Edge Down") -> (w455:T1)
      }
      frame "AccelCal: Display Front Edge Down" {
        n210 = Unbundle By Name(w470) -> ("Radians"=w479:dbl, "ModelRef"=w485:refnum<vi>)
        n211 = call <vilib>:"Clear Transformation.vi"("Object Refnum In"=w485) -> ("Object Refnum Out"=w478:refnum<vi>)  [unwired: 9 in, 1 out]
        n212 = Compound Arithmetic op=MULTIPLY(180.0 ("value"), w479) -> (w481:dbl)
        n213 = call "NextState.vi"("State"="AccelCal: Update Display", "Queue In"=w462) -> ("Queue Out"=w461:refnum<queue>)  [unwired: 8 in, 1 out]
        n214 = call <vilib>:"Rotate Object.vi"("Angle"=w481, "Axis"=cluster{"X":sgl, "Y":sgl, "Z":sgl} {"X"=0.0, "Y"=1.0, "Z"=0.0}, "Scene.Object In"=w478) -> ("Scene.Object Out"=w482:refnum<vi>)  [unwired: 7 in, 1 out]
        n215 = Compound Arithmetic op=MULTIPLY(-90.0 ("value"), w479) -> (w480:dbl)
        n216 = call <vilib>:"Rotate Object.vi"("Angle"=w480, "Axis"=cluster{"X":sgl, "Y":sgl, "Z":sgl} {"X"=1.0, "Y"=0.0, "Z"=0.0}, "Scene.Object In"=w482) -> ("Scene.Object Out"=w477:refnum<vi>)  [unwired: 7 in, 1 out]
        n217 = Compound Arithmetic op=MULTIPLY(0.0 ("value"), w479) -> (w475:dbl)
        n218 = call "NextState.vi"("State"="Response: Enable", "Queue In"=w461) -> ("Queue Out"=w465:refnum<queue>)  [unwired: 8 in, 1 out]
        n219 = call <vilib>:"Rotate Object.vi"("Angle"=w475, "Axis"=cluster{"X":sgl, "Y":sgl, "Z":sgl} {"X"=0.0, "Y"=0.0, "Z"=1.0}, "Scene.Object In"=w477) -> ("Scene.Object Out"=w474:refnum<vi>)  [unwired: 7 in, 1 out]
        n220 = Bundle By Name(cluster=w470, "NextState"="AccelCal: Wait Front Edge Down", "ModelRef"=w474) -> (w469:T1)
        n221 = call "NextState.vi"("Data"="Place the AeroQuad front edge down.  The arrow indicates the front of the AeroQuad." ("State"), "State"="Instructions: Update", "Queue In"=w465) -> ()  [unwired: 7 in, 2 out]
      }
      frame "AccelCal: Wait Front Edge Down" {
        n222 = call "NextState.vi"("Data"=TRUE, "State"="AccelCal: Request Telemetry", "Queue In"=w491) -> ()  [unwired: 7 in, 2 out]
        n223 = Bundle By Name(cluster=w489, "AccelRaw"=dbl[][] [], "AccelIndex"=0, "NextState"="AccelCal: Calculate Cal") -> (w488:T1)
      }
      frame "AccelCal: Update Display" {
        n224 = Unbundle By Name(w495) -> ("ModelRef"=→"AccelGUI":refnum<vi>)
      }
      frame "AccelCal: Update" {
        w497 = 100 ("y")
        # "x, y, z"
        n225 = Unbundle By Name(w505) -> ("NextState"=w500:string, "AccelIndex"=w499:i32, "Data"=w498:dbl[][], "AccelRaw"=w506:dbl[][], "AccelData"=w501:dbl[][])
        n226 = Greater?(x=w499, y=w497) -> (0:w507:bool)
        n227 = case shown="False" w507 {
          tunnel: w508 -> [w528 w540]
          tunnel: w498 -> [_ w545]
          tunnel: w506 -> [w521 w544]
          tunnel: [_ w542] -> w503
          tunnel: w499 -> [_ w539]
          tunnel: [_ w532] -> w502
          tunnel: w501 -> [w524 w541]
          tunnel: [w523 w541] -> w496
          tunnel: w500 -> [w522 _]
          tunnel: w497 -> [_ w529]
          frame True {
            n228 = Index Array(array=w521, index (col) #1=0 ("disabled index (col)"), index (col) #2=1 ("index (col)"), index (col) #3=2 ("index (col)")) -> (element #1=w517:dbl[], element #2=w516:dbl[], element #3=w515:dbl[])  [unwired: 3 in]
            n229 = call <vilib>:"Mean.vi"("X"=w517) -> ("mean"=w511:dbl)  [unwired: 1 out]
            n230 = call <vilib>:"Mean.vi"("X"=w515) -> ("mean"=w509:dbl)  [unwired: 1 out]
            n231 = call <vilib>:"Mean.vi"("X"=w516) -> ("mean"=w510:dbl)  [unwired: 1 out]
            n232 = Build Array(w511, w510, w509) -> (w514:dbl[])
            n233 = Build Array (concatenate)(w524, w514) -> (w523:dbl[][])
            n234 = call "NextState.vi"("Data"=FALSE, "State"="AccelCal: Request Telemetry", "Queue In"=w528) -> ("Queue Out"=w525:refnum<queue>)  [unwired: 7 in, 1 out]
            n235 = call "NextState.vi"("State"=w522, "Queue In"=w525) -> ("Queue Out"=w512:refnum<queue>)  [unwired: 8 in, 1 out]
            n236 = call "NextState.vi"("State"="Response: Enable", "Queue In"=w512) -> ()  [unwired: 8 in, 2 out]
          }
          frame False {
            n237 = Divide(x=w539, y=w529) -> (x/y=w538:dbl)
            n238 = Index Array(array=w545) -> (element=w543:dbl[])  [unwired: 2 in]
            n239 = Multiply(x=100.0, y=w538) -> (x*y=w535:dbl)
            n240 = Build Array (concatenate)(w544, w543) -> (w542:dbl[][])
            n241 = Format Into String(format string="Calibration... %d %", w535) -> (resulting string=w533:string)  [unwired: 2 in, 1 out]
            n242 = Increment(x=w539) -> (x+1=w532:i32)
            n243 = call "NextState.vi"("Data"=w533, "State"="Instructions: Update", "Queue In"=w540) -> ("Queue Out"=w530:refnum<queue>)  [unwired: 7 in, 1 out]
            n244 = Greater?(x=w532, y=w529) -> (0:w531:bool)
            n245 = case shown="True" w531 {
              tunnel: w530 -> [_ w551]
              frame False {
              }
              frame True {
                n246 = call "LookupCommands.vi"("CommandName"="StopTelem") -> ("CommandValue"=w546:string)  [unwired: 10 in]
                n247 = call "NextGUIState.vi"("GUI State"="Clear Queue" ("State"), "Queue In"=w551) -> ("Queue Out"=w549:refnum<queue>)  [unwired: 8 in, 1 out]
                n248 = call "NextGUIState.vi"("State Argument"=w546, "GUI State"="Request Telemetry" ("State"), "Queue In"=w549) -> ("Queue Out"=w548:refnum<queue>)  [unwired: 7 in, 1 out]
                n249 = call "NextGUIState.vi"("GUI State"="Clear Serial Comm" ("State"), "Queue In"=w548) -> ()  [unwired: 8 in, 2 out]
              }
            }
          }
        }
        n250 = Bundle By Name(cluster=w505, "AccelIndex"=w502, "AccelRaw"=w503, "AccelData"=w496) -> (w504:T1)
      }
      frame "AccelCal: Calculate Cal" {
        # "m = (upSideDown - rightSideUp)/(9.8065 - (-9.8065));\nzAxisAccelBias = upSideDown - m * 9.8065;\nbiased = upSideDown - zAxisAccelBias;\nzAxisAccelScaleFactor = 9.8065 / biased;"
        # "0 = x\n1 = y\n2 = z"
        # "0 - right side up\n1 - upside down\n2 - left down\n3 - right down\n4 - rear down\n5 - front down"
        n251 = Unbundle By Name(w555) -> ("AccelData"=w559:dbl[][])
        n252 = for {
          N: 3 -> [_]
          tunnel: w559 -> [w564]
          tunnel: [w566] -> w556 mode=indexing
          tunnel: [w565] -> w557 mode=indexing
          i -> [w562]
          n253 = case shown="1" w562 {
            tunnel: [5 ("index (row)") 3 ("index (row)") 0 ("index (row)")] -> w579
            tunnel: [0 ("disabled index (col)") 1 ("disabled index (col)") 2 ("disabled index (col)")] -> w578
            tunnel: [0 ("disabled index (col)") 1 ("disabled index (col)") 2 ("disabled index (col)")] -> w577
            tunnel: [4 ("index (row)") 2 ("index (row)") 1 ("index (row)")] -> w576
            tunnel: [w580 w585 w594] -> w563
            tunnel: w564 -> [w580 w585 w594]
            frame 0, Default {
            }
            frame 1 {
            }
            frame 2 {
            }
          }
          n254 = Index Array ("upsideDown")(array=w563, index (row)=w576, index (col)=w577) -> (element=w569:dbl)
          n255 = Index Array ("rightSideUp")(array=w563, index (row)=w579, index (col)=w578) -> (element=w575:dbl)
          n256 = Subtract(x=w569, y=w575) -> (x-y=w574:dbl)
          n257 = Divide "m"(x=w574, y=19.613) -> (x/y=w572:dbl)
          n258 = Multiply(x=w572, y=9.8065) -> (x*y=w570:dbl)
          n259 = Subtract "AccelBias"(x=w569, y=w570) -> (x-y=w566:dbl)
          n260 = Subtract "biased"(x=w569, y=w566) -> (x-y=w567:dbl)
          n261 = Divide "AccelScaleFactor"(x=9.8065 ("y"), y=w567) -> (x/y=w565:dbl)
        }
        n262 = call "NextState.vi"("State"="AccelCal: Generate Cal", "Queue In"=w560) -> ()  [unwired: 8 in, 2 out]
        n263 = Bundle By Name(cluster=w555, "AccelScaleFactor"=w557, "AccelBias"=w556) -> (w554:T1)
      }
      frame "AccelCal: Generate Cal" {
        w601 = "Send Command" ("State")
        n264 = Unbundle By Name(w613) -> ("AccelScaleFactor"=w617:dbl[], "AccelBias"=w618:dbl[])
        n265 = Interleave 1D Arrays(w617, w618) -> (w621:dbl[])
        n266 = call "NextState.vi"("State"="AccelCal: Reset Display", "Queue In"=w634) -> ("Queue Out"=w609:refnum<queue>)  [unwired: 8 in, 1 out]
        n267 = Number To Fractional String(number=w621, precision (6)=i16 6) -> (F-format string=w619:string[])  [unwired: 2 in]
        n268 = Array To Spreadsheet String(delimiter (Tab)=";", array=w619, 3:"%s" ("format string")) -> (spreadsheet string=w629:string)
        n269 = Match Pattern(string=w629, regular expression="\r\n") -> (before substring=w604:string)  [unwired: 4 out]
        n270 = call "LookupCommands.vi"("CommandName"="AccelCal") -> ("CommandValue"=w606:string)  [unwired: 10 in]
        n271 = Concatenate Strings(w606, w604, ";" ("string")) -> (w595:string)
        n272 = call "LookupCommands.vi"("CommandName"="WriteEPPROM") -> ("CommandValue"=w605:string)  [unwired: 10 in]
        n273 = call "NextState.vi"("State"="Response: OK Only", "Queue In"=w609) -> ("Queue Out"=w608:refnum<queue>)  [unwired: 8 in, 1 out]
        n274 = Bundle By Name(cluster=w613, "NextState"="AccelCal: Generate Accel Bias") -> (w612:T1)
        n275 = call "NextState.vi"("Data"="Return the AeroQuad to a level position.  Select OK to finalize and store the calibration." ("State"), "State"="Instructions: Update", "Queue In"=w608) -> ("Queue Out"=w614:refnum<queue>)  [unwired: 7 in, 1 out]
        n276 = call "NextGUIState.vi"("GUI State"="Clear Queue" ("State"), "Queue In"=w614) -> ("Queue Out"=w622:refnum<queue>)  [unwired: 8 in, 1 out]
        n277 = call "NextGUIState.vi"("GUI State"="Clear Serial Comm" ("State"), "Queue In"=w622) -> ("Queue Out"=w632:refnum<queue>)  [unwired: 8 in, 1 out]
        n278 = call "NextGUIState.vi"("State Argument"=w595, "GUI State"=w601, "Queue In"=w632) -> ("Queue Out"=w626:refnum<queue>)  [unwired: 7 in, 1 out]
        n279 = call "NextGUIState.vi"("GUI State"="Delay SubPanel", "Queue In"=w626) -> ("Queue Out"=w603:refnum<queue>)  [unwired: 8 in, 1 out]
        n280 = call "NextGUIState.vi"("State Argument"=w605, "GUI State"=w601, "Queue In"=w603) -> ("Queue Out"=w600:refnum<queue>)  [unwired: 7 in, 1 out]
        n281 = call "NextGUIState.vi"("State Argument"="1000", "GUI State"="Delay String" ("State"), "Queue In"=w600) -> ("Queue Out"=w597:refnum<queue>)  [unwired: 7 in, 1 out]
        n282 = call "NextGUIState.vi"("State Argument"=w595, "GUI State"="Store Calibration", "Queue In"=w597) -> ()  [unwired: 7 in, 2 out]
      }
      frame "AccelCal: Generate Accel Bias" {
        n283 = call "LookupCommands.vi"("CommandName"="AccelBias") -> ("CommandValue"=w645:string)  [unwired: 10 in]
        n284 = call "NextGUIState.vi"("State Argument"=w645, "GUI State"="Send Command", "Queue In"=w650) -> ("Queue Out"=w643:refnum<queue>)  [unwired: 7 in, 1 out]
        n285 = call "LookupCommands.vi"("CommandName"="WriteEPPROM") -> ("CommandValue"=w641:string)  [unwired: 10 in]
        n286 = call "NextGUIState.vi"("State Argument"=w641, "GUI State"="Send Command" ("State"), "Queue In"=w643) -> ("Queue Out"=w640:refnum<queue>)  [unwired: 7 in, 1 out]
        n287 = call "NextGUIState.vi"("State Argument"="1000", "GUI State"="Delay String", "Queue In"=w640) -> ("Queue Out"=w635:refnum<queue>)  [unwired: 7 in, 1 out]
        n288 = local write "Instruction"("Calibration Complete" ("Instruction")) -> ()
        n289 = call "NextGUIState.vi"("State Argument"="Accelerometer Calibration Complete" ("State"), "GUI State"="Status" ("State"), "Queue In"=w635) -> ()  [unwired: 7 in, 2 out]
      }
      frame "AccelCal: Reset Display" {
        n290 = Unbundle By Name(w655) -> ("Radians"=w656:dbl, "ModelRef"=w669:refnum<vi>)
        n291 = call <vilib>:"Clear Transformation.vi"("Object Refnum In"=w669) -> ("Object Refnum Out"=w657:refnum<vi>)  [unwired: 9 in, 1 out]
        n292 = Compound Arithmetic op=MULTIPLY(0.0 ("value"), w656) -> (w665:dbl)
        n293 = call "NextState.vi"("State"="AccelCal: Update Display", "Queue In"=w652) -> ()  [unwired: 8 in, 2 out]
        n294 = call <vilib>:"Rotate Object.vi"("Angle"=w665, "Axis"=cluster{"X":sgl, "Y":sgl, "Z":sgl} {"X"=0.0, "Y"=1.0, "Z"=0.0}, "Scene.Object In"=w657) -> ("Scene.Object Out"=w666:refnum<vi>)  [unwired: 7 in, 1 out]
        n295 = Compound Arithmetic op=MULTIPLY(0.0 ("value"), w656) -> (w664:dbl)
        n296 = call <vilib>:"Rotate Object.vi"("Angle"=w664, "Axis"=cluster{"X":sgl, "Y":sgl, "Z":sgl} {"X"=1.0, "Y"=0.0, "Z"=0.0}, "Scene.Object In"=w666) -> ("Scene.Object Out"=w663:refnum<vi>)  [unwired: 7 in, 1 out]
        n297 = Compound Arithmetic op=MULTIPLY(0.0 ("value"), w656) -> (w661:dbl)
        n298 = call <vilib>:"Rotate Object.vi"("Angle"=w661, "Axis"=cluster{"X":sgl, "Y":sgl, "Z":sgl} {"X"=0.0, "Y"=0.0, "Z"=1.0}, "Scene.Object In"=w663) -> ("Scene.Object Out"=w653:refnum<vi>)  [unwired: 7 in, 1 out]
        n299 = Bundle By Name(cluster=w655, "ModelRef"=w653) -> (w654:T1)
      }
      frame "TransmitterCal: Hide", "TransmitterCal: Show" {
        n300 = property class="VI"() -> ("Panel"=w672:refnum<vi>)  [unwired: 2 in, 2 out]
        n301 = Match Pattern(string=w676, regular expression="Show") -> (offset past match=w674:i32)  [unwired: 1 in, 3 out]
        n302 = Greater Or Equal To 0?(x=w674) -> (x >= 0?=w671:bool)
        n303 = property class="Pnl"(reference=w672) -> ("Controls[]"=w673:refnum<vi>[])  [unwired: 1 in, 2 out]
        n304 = for {
          tunnel: w673 -> [w683] mode=indexing
          tunnel: w671 -> [w681]
          tunnel: string[] ["Left Stick", "Right Stick", "Throttle", "ThrottleBar", "Yaw", "YawBar", "Roll", "RollBar", "Pitch", "PitchBar", "Mode", "ModeBar", "AUX1", "AUX1Bar", "AUX2", "AUX2Bar", "AUX3", "AUX3Bar"] -> [w680]
          n305 = property class="Ctl"(reference=w683) -> (reference out=w682:refnum<vi>, "Label.Text"=w679:string)  [unwired: 1 in, 1 out]
          n306 = Search 1D Array(1D array=w680, element=w679) -> (index of element=w678:i32)  [unwired: 1 in]
          n307 = case shown="0.." w678 {
            tunnel: w682 -> [_ w685]
            tunnel: w681 -> [_ w684]
            frame Default {
            }
            frame 0.. {
              n308 = property class="Ctl"(reference=w685, "Visible"=w684) -> ()  [unwired: 1 in, 2 out]
            }
          }
        }
      }
      frame "TransmitterCal: Update Channels" {
        n309 = Unbundle By Name(w697) -> ("SubPanelData"=w688:string[][])
        n310 = Index Array(array=w688, index (col)=0 ("index (row)")) -> (element=w693:string[])  [unwired: 1 in]
        n311 = call "NextState.vi"("State"="TransmitterCal: Start Cal", "Queue In"=w695) -> ()  [unwired: 8 in, 2 out]
        n312 = Search 1D Array(1D array=w693, element="Receiver Channels") -> (index of element=w690:i32)  [unwired: 1 in]
        n313 = Index Array(array=w688, index (row)=w690, index (col)=1 ("disabled index (col)")) -> (element=w687:string)
        n314 = Decimal String To Number(string=w687) -> (number=w686:i32)  [unwired: 2 in, 1 out]
        n315 = Bundle By Name(cluster=w697, "XmitCount"=w686) -> (w696:T1)
      }
      frame "TransmitterCal: Start Cal" {
        n316 = flat-sequence {
          tunnel: w699 -> [w733]
          tunnel: [w733] -> w698
          frame #0 {
            n317 = One Button Dialog(message="Verify transmitter is turned on and connection established to the receiver.") -> ()  [unwired: 1 in, 1 out]
          }
          frame #1 {
            n318 = One Button Dialog(message="Before starting the calibration, set the transmitter to it's default settings.  It can be in Airplane or Helicopter mode.\n\nVerify that:\n- ESC's and motors are disconnected from power! \n- Trims and subtrims are zero\n- Travel Adjust / End Point Adjustment (EPA) are 100%\n\nStep 1:  Check that the transmitter sticks move in the same direction as on the Transmitter Adjustment screen.  If any channels move backwards, use the channel reversing function on your transmitter to make the direction match. Example: If the pitch stick is moved up, the pitch indicator in the Configurator should move up as well, not down.\n\nStep 2: For Futaba users only - Manually set the EPA for Mode (typically channel 5) and Aux (typically channel 6) to 50% at both the maximum and minimum ends.\n\nStep 3: Move both transmitter sticks to each of it's four corners (upper left, upper right, lower left, lower right). Wait a second or two at each extreme to be sure to capture the farthest position.\n\nStep 4: Flip any transmitter switches assigned to Mode or Aux to all positions. (If your transmitter is setup in Helicopter Mode, it is normal that the Aux channel moves with the Throttle channel.  If you want to customize the code to assign the Aux channel to a switch, configure your transmitter for Airplane Mode.\n\nPress NEXT when ready to begin calibration.", button name ("OK")="Next") -> ()  [unwired: 1 out]
          }
        }
        n319 = Unbundle By Name(w698) -> ("XmitCount"=w723:i32)
        n320 = call "NextGUIState.vi"("GUI State"="Clear Queue", "Queue In"=w726) -> ("Queue Out"=w724:refnum<queue>)  [unwired: 8 in, 1 out]
        n321 = call "NextGUIState.vi"("GUI State"="Clear Serial Comm", "Queue In"=w724) -> ("Queue Out"=w701:refnum<queue>)  [unwired: 8 in, 1 out]
        n322 = call "LookupCommands.vi"("CommandName"="TransmitterTelem") -> ("CommandValue"=w711:string)  [unwired: 10 in]
        n323 = call "LookupCommands.vi"("CommandName"="TransmitterSlope") -> ("CommandValue"=w722:string)  [unwired: 10 in]
        n324 = call "LookupCommands.vi"("CommandName"="TransmitterOffset") -> ("CommandValue"=w721:string)  [unwired: 10 in]
        n325 = call "NextGUIState.vi"("State Argument"="Setting transmitter calibration to default values...", "GUI State"="Status", "Queue In"=w701) -> ("Queue Out"=w700:refnum<queue>)  [unwired: 7 in, 1 out]
        n326 = for {
          N: w723 -> [_]
          tunnel: w722 -> [w754]
          tunnel: w721 -> [w755]
          tunnel: w700 -> [w751]
          tunnel: [0.0] -> w718 mode=indexing
          tunnel: [3000.0] -> w717 mode=indexing
          tunnel: [w739] -> w704
          i -> [w752]
          w744 = "Delay String" ("State")
          w747 = "Send Command" ("State")
          w753 = "%d;%f;" ("format string")
          n327 = Format Into String(format string=w753, initial string=w755, w752, 0.0) -> (resulting string=w743:string)  [unwired: 1 in, 1 out]
          n328 = call "NextGUIState.vi"("State Argument"=w743, "GUI State"=w747, "Queue In"=w751) -> ("Queue Out"=w750:refnum<queue>)  [unwired: 7 in, 1 out]
          n329 = Format Into String(format string=w753, initial string=w754, w752, 1.0) -> (resulting string=w742:string)  [unwired: 1 in, 1 out]
          n330 = call "NextGUIState.vi"("State Argument"="50", "GUI State"=w744, "Queue In"=w750) -> ("Queue Out"=w748:refnum<queue>)  [unwired: 7 in, 1 out]
          n331 = call "NextGUIState.vi"("State Argument"=w742, "GUI State"=w747, "Queue In"=w748) -> ("Queue Out"=w745:refnum<queue>)  [unwired: 7 in, 1 out]
          n332 = call "NextGUIState.vi"("State Argument"="50", "GUI State"=w744, "Queue In"=w745) -> ("Queue Out"=w739:refnum<queue>)  [unwired: 7 in, 1 out]
        }
        n333 = call "NextGUIState.vi"("State Argument"=w711, "GUI State"="Send Command" ("State"), "Queue In"=w704) -> ("Queue Out"=w716:refnum<queue>)  [unwired: 7 in, 1 out]
        n334 = call "NextGUIState.vi"("GUI State"="Read Continuous" ("State"), "Queue In"=w716) -> ("Queue Out"=w715:refnum<queue>)  [unwired: 8 in, 1 out]
        n335 = call "NextState.vi"("State"="Response: Enable", "Queue In"=w715) -> ("Queue Out"=w707:refnum<queue>)  [unwired: 8 in, 1 out]
        n336 = call "NextState.vi"("Data"="Move the transmitter sticks and switches to their maximum and minimum values.  Press OK when calibration is complete.  To abort press Cancel." ("State"), "State"="Instructions: Update", "Queue In"=w707) -> ("Queue Out"=w706:refnum<queue>)  [unwired: 7 in, 1 out]
        n337 = Bundle By Name(cluster=w699, "TlmType"="TransmitterCal: Update", "Response"=enum16{"Wait", "OK", "Cancel"}."Wait", "NextState"="TransmitterCal: Generate Cal") -> (w720:T1)
        n338 = Bundle By Name(cluster=w720, "XmitMax"=w718, "XmitMin"=w717) -> (w719:T1)
        n339 = call "NextState.vi"("State"="TransmitterCal: Initialize Graphics", "Queue In"=w706) -> ()  [unwired: 8 in, 2 out]
      }
      frame "TransmitterCal: Initialize Graphics" {
        w768 = "TxCalDial.png" ("File")
        n340 = Unbundle By Name(w774) -> ("WorkingFolder"=w759:path)
        n341 = call <vilib>:"Create Sphere.vi"("Detail"=sgl 1.0, "Color"=T4 {"Red"=0.0, "Green"=0.0, "Blue"=1.0, "Alpha"=1.0}, "Radius"=sgl 0.25) -> ("New Sphere Refnum"=w779:refnum<vi>)  [unwired: 1 in, 7 out]
        n342 = call <vilib>:"Create Object.vi"("Name"="Right") -> ("Scene:New Object"=w784:refnum<vi>)  [unwired: 9 in, 1 out]
        n343 = call <vilib>:"Create Sphere.vi"("Detail"=sgl 1.0, "Color"=T4 {"Red"=0.0, "Green"=0.0, "Blue"=1.0, "Alpha"=1.0}, "Radius"=sgl 0.25) -> ("New Sphere Refnum"=w783:refnum<vi>)  [unwired: 1 in, 7 out]
        n344 = call <vilib>:"Create Object.vi"("Name"="Left") -> ("Scene:New Object"=w786:refnum<vi>)  [unwired: 9 in, 1 out]
        n345 = invoke class="SceneObject" method="Set Drawable"(reference=w784, "Drawable"=w779) -> (reference out=w776:refnum<vi>)  [unwired: 2 in, 3 out]
        n346 = invoke class="SceneObject" method="Set Drawable"(reference=w786, "Drawable"=w783) -> (reference out=w766:refnum<vi>)  [unwired: 2 in, 3 out]
        n347 = call "ViewWindowCreate.vi"("File"=w768, "Solid Horizon Path.PNG"=w759) -> ("SceneObject out"=w773:refnum<vi>)  [unwired: 9 in]
        n348 = call "ViewWindowCreate.vi"("File"=w768, "Solid Horizon Path.PNG"=w759) -> ("SceneObject out"=w764:refnum<vi>)  [unwired: 9 in]
        n349 = call "NextGUIState.vi"("State Argument"="Performing transmitter calibration...", "GUI State"="Status", "Queue In"=w756) -> ()  [unwired: 7 in, 2 out]
        n350 = property class="SceneObject"(reference=w766, "Specials.Texturing"=enum16{"Inherit Value", "Off", "On"}."Off" ("Specials:Texturing")) -> (reference out=w765:refnum<vi>)  [unwired: 1 in, 1 out]
        n351 = property class="SceneObject"(reference=w776, "Specials.Texturing"=enum16{"Inherit Value", "Off", "On"}."Off" ("Specials:Texturing")) -> (reference out=w775:refnum<vi>)  [unwired: 1 in, 1 out]
        n352 = invoke class="SceneObject" method="Object.Add Object"(reference=w764, "Child"=w765) -> (reference out=w762:refnum<vi>, "Child"=w760:refnum<vi>)  [unwired: 2 in, 2 out]
        n353 = invoke class="SceneObject" method="Object.Add Object"(reference=w773, "Child"=w775) -> (reference out=w771:refnum<vi>, "Child"=w769:refnum<vi>)  [unwired: 2 in, 2 out]
        n354 = call <vilib>:"Translate Object.vi"("Translation"=cluster{"X":sgl, "Y":sgl, "Z":sgl} {"X"=0.0, "Y"=0.0, "Z"=1.0}, "Scene.Object In"=w762) -> ("Scene.Object Out"=w761:refnum<vi>)  [unwired: 8 in, 1 out]
        n355 = call <vilib>:"Translate Object.vi"("Translation"=cluster{"X":sgl, "Y":sgl, "Z":sgl} {"X"=0.0, "Y"=0.0, "Z"=1.0}, "Scene.Object In"=w771) -> ("Scene.Object Out"=w770:refnum<vi>)  [unwired: 8 in, 1 out]
        n356 = Bundle By Name(cluster=w774, "RightStickScene"=w770, "RightStick"=w769, "LeftStick"=w760, "LeftStickScene"=w761) -> (w790:T1)
      }
      frame "TransmitterCal: Update" {
        w819 = 0 ("index (row)")
        w824 = 0 ("index (row)")
        n357 = Unbundle By Name(w826) -> ("LeftStick"=w793:refnum<vi>, "RightStick"=w798:refnum<vi>, "Data"=w815:dbl[][])
        n358 = Index Array(array=w815, index (row) #1=w824, index (col) #1=0 ("disabled index (col)"), index (row) #2=w824, index (col) #2=1 ("disabled index (col)"), index (row) #3=w824, index (col) #3=2 ("disabled index (col)"), index (row) #4=w824, index (col) #4=3 ("disabled index (col)")) -> (element #1=w795:dbl, element #2=w794:dbl, element #3=w797:dbl, element #4=w796:dbl)
        "ThrottleBar" <- w796
        "Throttle" <- w796
        "Roll" <- w795
        "RollBar" <- w795
        "Pitch" <- w794
        "PitchBar" <- w794
        "Yaw" <- w797
        "YawBar" <- w797
        n359 = call "NextState.vi"("State"="TransmitterCal: Max/Min", "Queue In"=w792) -> ()  [unwired: 8 in, 2 out]
        n360 = expression code="(0.002*x) - 3"(w797) -> (w809:dbl)
        n361 = expression code="(0.002*x) - 3"(w796) -> (w810:dbl)
        n362 = call <vilib>:"Clear Transformation.vi"("Object Refnum In"=w793) -> ("error out"=w805:errorcluster, "Object Refnum Out"=w806:refnum<vi>)  [unwired: 9 in]
        n363 = expression code="(0.002*x) - 3"(w795) -> (w803:dbl)
        n364 = expression code="(0.002*x) - 3"(w794) -> (w804:dbl)
        n365 = Bundle By Name(cluster=cluster{"X":sgl, "Y":sgl, "Z":sgl} {"X"=0.0, "Y"=0.0, "Z"=0.0} ("Translation"), "X"=w809, "Y"=w810) -> (w808:cluster{"X":sgl, "Y":sgl, "Z":sgl})
        n366 = call <vilib>:"Translate Object.vi"("error in (no error)"=w805, "Translation"=w808, "Scene.Object In"=w806) -> ()  [unwired: 7 in, 2 out]
        n367 = call <vilib>:"Clear Transformation.vi"("Object Refnum In"=w798) -> ("error out"=w799:errorcluster, "Object Refnum Out"=w800:refnum<vi>)  [unwired: 9 in]
        n368 = Index Array(array=w815, index (row) #1=w819, index (col) #1=4 ("disabled index (col)"), index (row) #2=w819, index (col) #2=5 ("disabled index (col)"), index (row) #3=w819, index (col) #3=6 ("disabled index (col)"), index (row) #4=w819, index (col) #4=7 ("disabled index (col)")) -> (element #1=→"Mode" →"ModeBar":dbl, element #2=→"AUX1" →"AUX1Bar":dbl, element #3=→"AUX2Bar" →"AUX2":dbl, element #4=→"AUX3" →"AUX3Bar":dbl)
        n369 = Bundle By Name(cluster=cluster{"X":sgl, "Y":sgl, "Z":sgl} {"X"=0.0, "Y"=0.0, "Z"=0.0} ("Translation"), "X"=w803, "Y"=w804) -> (w802:cluster{"X":sgl, "Y":sgl, "Z":sgl})
        n370 = call <vilib>:"Translate Object.vi"("error in (no error)"=w799, "Translation"=w802, "Scene.Object In"=w800) -> ()  [unwired: 7 in, 2 out]
      }
      frame "TransmitterCal: Max/Min" {
        n371 = Unbundle By Name(w834) -> ("LeftStickScene"=→"Left Stick":refnum<vi>, "RightStickScene"=→"Right Stick":refnum<vi>, "XmitMax"=w836:dbl[], "XmitMin"=w835:dbl[], "Data"=w831:dbl[][])
        n372 = Index Array(array=w831, index (row)=0 ("disabled index (col)")) -> (element=w837:dbl[])  [unwired: 1 in]
        n373 = for {
          tunnel: w837 -> [w839] mode=indexing
          tunnel: w836 -> [w842] mode=indexing
          tunnel: w835 -> [w840] mode=indexing
          tunnel: [w841] -> w830 mode=indexing
          tunnel: [w838] -> w829 mode=indexing
          n374 = Max & Min(x=w842, y=w839) -> (max(x,y)=w841:dbl)  [unwired: 1 out]
          n375 = Max & Min(x=w840, y=w839) -> (min(x,y)=w838:dbl)  [unwired: 1 out]
        }
        n376 = Bundle By Name(cluster=w834, "XmitMax"=w830, "XmitMin"=w829) -> (w833:T1)
      }
      frame "TransmitterCal: Generate Cal" {
        w849 = "Delay String" ("State")
        w855 = "Verify Upload" ("State")
        n377 = Unbundle By Name(w882) -> ("XmitMax"=w885:dbl[], "XmitMin"=w884:dbl[], "XmitCount"=w883:i32)
        n378 = call "NextGUIState.vi"("GUI State"="Clear Queue", "Queue In"=w886) -> ("Queue Out"=w888:refnum<queue>)  [unwired: 8 in, 1 out]
        n379 = call "GenerateTransmitterCal.vi"("XmitCount"=w883, "XmitMin"=w884, "XmitMax"=w885) -> ("TransmitterSlopeFloat"=w876:dbl[], "TransmitterOffsetFloat"=w877:dbl[], "TransmitterOffset"=w860:string[], "TransmitterSlope"=w856:string[])  [unwired: 5 in]
        n380 = call "LookupCommands.vi"("CommandName"="TransmitterSlope") -> ("CommandValue"=w879:string)  [unwired: 10 in]
        n381 = call "LookupCommands.vi"("CommandName"="TransmitterOffset") -> ("CommandValue"=w878:string)  [unwired: 10 in]
        n382 = call "NextGUIState.vi"("GUI State"="Clear Serial Comm" ("State"), "Queue In"=w888) -> ("Queue Out"=w846:refnum<queue>)  [unwired: 8 in, 1 out]
        n383 = call "NextGUIState.vi"("State Argument"="Storing transmitter calibration...", "GUI State"="Status", "Queue In"=w846) -> ("Queue Out"=w845:refnum<queue>)  [unwired: 7 in, 1 out]
        n384 = for {
          tunnel: w879 -> [w908]
          tunnel: w878 -> [w909]
          tunnel: w877 -> [w906] mode=indexing
          tunnel: w876 -> [w905] mode=indexing
          tunnel: w845 -> [w903]
          tunnel: [w893] -> w864
          i -> [w904]
          w892 = "Store Calibration" ("GUI State")
          w896 = "Delay String" ("State")
          w899 = "Send Command" ("State")
          w907 = "%d;%f;" ("format string")
          n385 = Format Into String(format string=w907, initial string=w909, w904, w906) -> (resulting string=w891:string)  [unwired: 1 in, 1 out]
          n386 = call "NextGUIState.vi"("State Argument"=w891, "GUI State"=w899, "Queue In"=w903) -> ("Queue Out"=w902:refnum<queue>)  [unwired: 7 in, 1 out]
          n387 = Format Into String(format string=w907, initial string=w908, w904, w905) -> (resulting string=w890:string)  [unwired: 1 in, 1 out]
          n388 = call "NextGUIState.vi"("State Argument"="50", "GUI State"=w896, "Queue In"=w902) -> ("Queue Out"=w900:refnum<queue>)  [unwired: 7 in, 1 out]
          n389 = call "NextGUIState.vi"("State Argument"=w890, "GUI State"=w899, "Queue In"=w900) -> ("Queue Out"=w897:refnum<queue>)  [unwired: 7 in, 1 out]
          n390 = call "NextGUIState.vi"("State Argument"="50", "GUI State"=w896, "Queue In"=w897) -> ("Queue Out"=w895:refnum<queue>)  [unwired: 7 in, 1 out]
          n391 = call "NextGUIState.vi"("State Argument"=w891, "GUI State"=w892, "Queue In"=w895) -> ("Queue Out"=w894:refnum<queue>)  [unwired: 7 in, 1 out]
          n392 = call "NextGUIState.vi"("State Argument"=w890, "GUI State"=w892, "Queue In"=w894) -> ("Queue Out"=w893:refnum<queue>)  [unwired: 7 in, 1 out]
        }
        n393 = call "LookupCommands.vi"("CommandName"="TransmitterOffsetResponse") -> ("CommandValue"=w861:string)  [unwired: 10 in]
        n394 = call "LookupCommands.vi"("CommandName"="TransmitterSlopeResponse") -> ("CommandValue"=w857:string)  [unwired: 10 in]
        n395 = call "LookupCommands.vi"("CommandName"="TransmitterTelem") -> ("CommandValue"=w869:string)  [unwired: 10 in]
        n396 = call "NextGUIState.vi"("State Argument"=w861, "GUI State"="Send Command" ("State"), "Queue In"=w864) -> ("Queue Out"=w863:refnum<queue>)  [unwired: 7 in, 1 out]
        n397 = call "ConvertCmd2TlmArguments.vi"("Input Command Arg"=w860) -> ("Output Telem Arg"=w867:string)  [unwired: 4 in]
        n398 = call "NextGUIState.vi"("State Argument"=w867, "GUI State"=w855, "Queue In"=w863) -> ("Queue Out"=w853:refnum<queue>)  [unwired: 7 in, 1 out]
        n399 = call "NextGUIState.vi"("State Argument"="250", "GUI State"=w849, "Queue In"=w853) -> ("Queue Out"=w852:refnum<queue>)  [unwired: 7 in, 1 out]
        n400 = call "NextGUIState.vi"("State Argument"=w857, "GUI State"="Send Command" ("State"), "Queue In"=w852) -> ("Queue Out"=w859:refnum<queue>)  [unwired: 7 in, 1 out]
        n401 = call "ConvertCmd2TlmArguments.vi"("Input Command Arg"=w856) -> ("Output Telem Arg"=w858:string)  [unwired: 4 in]
        n402 = call "NextGUIState.vi"("State Argument"=w858, "GUI State"=w855, "Queue In"=w859) -> ("Queue Out"=w850:refnum<queue>)  [unwired: 7 in, 1 out]
        n403 = call "NextGUIState.vi"("State Argument"="250", "GUI State"=w849, "Queue In"=w850) -> ("Queue Out"=w847:refnum<queue>)  [unwired: 7 in, 1 out]
        n404 = call "NextGUIState.vi"("State Argument"=w869, "GUI State"="Send Command" ("State"), "Queue In"=w847) -> ("Queue Out"=w875:refnum<queue>)  [unwired: 7 in, 1 out]
        n405 = call "NextGUIState.vi"("GUI State"="Read Continuous" ("State"), "Queue In"=w875) -> ("Queue Out"=w870:refnum<queue>)  [unwired: 8 in, 1 out]
        n406 = call "NextState.vi"("Data"="Transmitter calibration values sent to AeroQuad.  Verify that all values go between 1000 - 2000.  If not, perform the calibration again." ("State"), "State"="Instructions: Update", "Queue In"=w870) -> ()  [unwired: 7 in, 2 out]
      }
      frame "ESCCal: Start Cal" {
        n407 = Two Button Dialog(message="Disconnect battery power NOW to the ESC's and motors before the start of the calibration.  Leave USB power ON to the AeroQuad.  Serious injury may occur if this step is not followed!", 1:"Abort" ("F button name (\"Cancel\")"), 2:"Battery Power Removed" ("T button name (\"OK\")")) -> (T button?=w914:bool)
        n408 = case shown="True" w914 {
          tunnel: w910 -> [w918 w921]
          frame False {
            n409 = call "NextState.vi"("Data"="ESC Calibration has been aborted.", "State"="LargeInstructions: Update", "Queue In"=w918) -> ()  [unwired: 7 in, 2 out]
          }
          frame True {
            n410 = call "NextState.vi"("State"="Response: Enable", "Queue In"=w921) -> ("Queue Out"=w925:refnum<queue>)  [unwired: 8 in, 1 out]
            n411 = call "NextState.vi"("Data"="Apply battery power to the ESC's and motors, then quickly hit OK." ("message"), "State"="Instructions: Update", "Queue In"=w925) -> ("Queue Out"=w924:refnum<queue>)  [unwired: 7 in, 1 out]
            n412 = call "NextState.vi"("Data"="This calibration process is for the Turnigy ESC's only.  This may work with other ESC's, consult the manufacturer's manual.\n\nWarning! Before starting this calibration, remove the propellers for safety considerations!  If this calibration is performed incorrectly, it could result in property damage and personal injury, as part of this calibration sends a high throttle command to the ESC's.\n\nWhat to expect: You should hear 2 short beeps when the high throttle position is being calibrated.  Then you wll hear 3 short beeps followed by 1 long beep once the low throttle position is calibrated.", "State"="LargeInstructions: Update", "Queue In"=w924) -> ()  [unwired: 7 in, 2 out]
          }
        }
        n413 = Bundle By Name(cluster=w913, "NextState"="ESCCal: High Throttle" ("State")) -> (w912:T1)
      }
      frame "ESCCal: High Throttle" {
        w940 = "LargeInstructions: Add Update" ("State")
        n414 = flat-sequence {
          tunnel: [w949] -> w943
          tunnel: w944 -> [w949]
          frame #0 {
            n415 = local read "LargeInstructions"() -> (w952:string)
            n416 = Concatenate Strings(w952, "\n\n**********\n\nStarting ESC Calibration" ("string")) -> (w951:string)
            n417 = local write "LargeInstructions"(w951) -> ()
          }
        }
        n418 = call "LookupCommands.vi"("CommandName"="ESCCalHigh") -> ("CommandValue"=w933:string)  [unwired: 10 in]
        n419 = call "NextGUIState.vi"("State Argument"=w933, "GUI State"="Send Command" ("State"), "Queue In"=w943) -> ("Queue Out"=w932:refnum<queue>)  [unwired: 7 in, 1 out]
        n420 = call "NextState.vi"("Data"="Starting High Throttle Calibration" ("Connection Status"), "State"=w940, "Queue In"=w932) -> ("Error Out"=w939:errorcluster, "Queue Out"=w937:refnum<queue>)  [unwired: 7 in]
        n421 = call "LookupCommands.vi"("CommandName"="ESCCalDelay") -> ("CommandValue"=w930:string)  [unwired: 10 in]
        n422 = Decimal String To Number(string=w930) -> (number=w929:i32)  [unwired: 2 in, 1 out]
        n423 = call "NextState.vi"("Error In"=w939, "Data"=w929, "State"="Delay", "Queue In"=w937) -> ("Error Out"=w938:errorcluster, "Queue Out"=w936:refnum<queue>)  [unwired: 6 in]
        n424 = call "NextState.vi"("Error In"=w938, "Data"="Completed High Throttle Calibration" ("State"), "State"=w940, "Queue In"=w936) -> ("Queue Out"=w946:refnum<queue>)  [unwired: 6 in, 1 out]
        n425 = call "NextState.vi"("State"="ESCCal: Low Throttle", "Queue In"=w946) -> ()  [unwired: 8 in, 2 out]
      }
      frame "ESCCal: Low Throttle" {
        w965 = "LargeInstructions: Add Update" ("State")
        n426 = call "LookupCommands.vi"("CommandName"="ESCCalLow") -> ("CommandValue"=w956:string)  [unwired: 10 in]
        n427 = call "NextGUIState.vi"("State Argument"=w956, "GUI State"="Send Command" ("State"), "Queue In"=w968) -> ("Queue Out"=w963:refnum<queue>)  [unwired: 7 in, 1 out]
        n428 = call "NextState.vi"("Data"="Starting Low Throttle Calibration" ("Connection Status"), "State"=w965, "Queue In"=w963) -> ("Error Out"=w960:errorcluster, "Queue Out"=w961:refnum<queue>)  [unwired: 7 in]
        n429 = call "LookupCommands.vi"("CommandName"="ESCCalDelay") -> ("CommandValue"=w954:string)  [unwired: 10 in]
        n430 = Decimal String To Number(string=w954) -> (number=w953:i32)  [unwired: 2 in, 1 out]
        n431 = call "NextState.vi"("Error In"=w960, "Data"=w953, "State"="Delay", "Queue In"=w961) -> ("Error Out"=w958:errorcluster, "Queue Out"=w959:refnum<queue>)  [unwired: 6 in]
        n432 = call "NextState.vi"("Error In"=w958, "Data"="Completed Low Throttle Calibration" ("State"), "State"=w965, "Queue In"=w959) -> ("Queue Out"=w966:refnum<queue>)  [unwired: 6 in, 1 out]
        n433 = call "NextState.vi"("State"="ESCCal: Check Motors", "Queue In"=w966) -> ()  [unwired: 8 in, 2 out]
      }
      frame "ESCCal: Check Motors" {
        w972 = ";" ("string")
        n434 = call "LookupCommands.vi"("CommandName"="ESCCheck") -> ("CommandValue"=w973:string)  [unwired: 10 in]
        n435 = call "LookupCommands.vi"("CommandName"="ESCCalMinValue") -> ("CommandValue"=w974:string)  [unwired: 10 in]
        n436 = Concatenate Strings(w973, w972, w974, w972) -> (w976:string)
        n437 = call "NextGUIState.vi"("State Argument"=w976, "GUI State"="Send Command" ("State"), "Queue In"=w983) -> ("Queue Out"=w977:refnum<queue>)  [unwired: 7 in, 1 out]
        n438 = call "NextState.vi"("State"="Response: OK Only", "Queue In"=w977) -> ("Queue Out"=w985:refnum<queue>)  [unwired: 8 in, 1 out]
        n439 = Bundle By Name(cluster=w990, "NextState"="ESCCal: Cal Finished") -> (w989:T1)
        n440 = call "NextState.vi"("Data"="Are all the motors spinning at the same rate?  If not, perform the calibration again." ("message"), "State"="Instructions: Update", "Queue In"=w985) -> ("Queue Out"=w980:refnum<queue>)  [unwired: 7 in, 1 out]
        n441 = call "NextState.vi"("Data"="Sending Test Motor Commands" ("State"), "State"="LargeInstructions: Add Update", "Queue In"=w980) -> ()  [unwired: 7 in, 2 out]
      }
      frame "ESCCal: Cal Finished" {
        n442 = call "LookupCommands.vi"("CommandName"="ESCCalOff") -> ("CommandValue"=w992:string)  [unwired: 10 in]
        n443 = Concatenate Strings(w992, ";1000;" ("string")) -> (w991:string)
        n444 = call "NextGUIState.vi"("State Argument"=w991, "GUI State"="Send Command" ("State"), "Queue In"=w1002) -> ("Queue Out"=w1001:refnum<queue>)  [unwired: 7 in, 1 out]
        n445 = local write "Instruction"("" ("Instruction")) -> ()
        n446 = call "NextGUIState.vi"("State Argument"="ESC Calibration Complete" ("Connection Status"), "GUI State"="Status" ("State"), "Queue In"=w1001) -> ("Queue Out"=w998:refnum<queue>)  [unwired: 7 in, 1 out]
        n447 = call "NextState.vi"("Data"="ESC Calibration Completed" ("State"), "State"="LargeInstructions: Add Update", "Queue In"=w998) -> ("Queue Out"=w997:refnum<queue>)  [unwired: 7 in, 1 out]
        n448 = call "NextState.vi"("State"="Response: Disable", "Queue In"=w997) -> ()  [unwired: 8 in, 2 out]
      }
      frame "MagnetometerCal: Hide", "MagnetometerCal: Show" {
        n449 = Match Pattern(string=w1009, regular expression="Show") -> (offset past match=w1011:i32)  [unwired: 1 in, 3 out]
        n450 = Greater Or Equal To 0?(x=w1011) -> (x >= 0?=w1007:bool)
        n451 = property on="X Axis" class="Slide (strict)"("Visible"=w1007) -> ()  [unwired: 2 in, 2 out]
        n452 = property on="Y Axis" class="Slide (strict)"("Visible"=w1007) -> ()  [unwired: 2 in, 2 out]
        n453 = property on="Z Axis" class="Slide (strict)"("Visible"=w1007) -> ()  [unwired: 2 in, 2 out]
      }
      frame "MagnetometerCal: Start Cal" {
        w1017 = cluster{dbl, dbl, dbl} {0.0, 0.0, 0.0} ("Y Axis")
        n454 = for {
          N: 3 -> [_]
          tunnel: [-1000.0] -> w1024 mode=indexing
          tunnel: [1000.0] -> w1023 mode=indexing
        }
        n455 = call "NextState.vi"("State"="Response: Enable", "Queue In"=w1030) -> ("Queue Out"=w1031:refnum<queue>)  [unwired: 8 in, 1 out]
        n456 = call "LookupCommands.vi"("CommandName"="MagTelem") -> ("CommandValue"=w1015:string)  [unwired: 10 in]
        n457 = Bundle By Name(cluster=w1025, "TlmType"="MagnetometerCal: Update", "MagMax"=w1024, "MagMin"=w1023, "NextState"="MagnetometerCal: Generate Cal") -> (w1021:T1)
        n458 = call "NextState.vi"("Data"="Rotate the AeroQuad along each axis multiple times.  Press OK when the calibration is complete.  To abort press Cancel." ("State"), "State"="Instructions: Update", "Queue In"=w1031) -> ("Queue Out"=w1029:refnum<queue>)  [unwired: 7 in, 1 out]
        n459 = call "NextGUIState.vi"("GUI State"="Clear Serial Comm", "Queue In"=w1029) -> ("Queue Out"=w1019:refnum<queue>)  [unwired: 8 in, 1 out]
        n460 = call "NextGUIState.vi"("State Argument"=w1015, "GUI State"="Send Command" ("State"), "Queue In"=w1019) -> ("Queue Out"=w1026:refnum<queue>)  [unwired: 7 in, 1 out]
        n461 = call "NextGUIState.vi"("GUI State"="Read Continuous" ("State"), "Queue In"=w1026) -> ("Queue Out"=w1012:refnum<queue>)  [unwired: 8 in, 1 out]
        n462 = call "NextGUIState.vi"("State Argument"="Performing Magnetometer Calibration" ("State"), "GUI State"="Status" ("State"), "Queue In"=w1012) -> ()  [unwired: 7 in, 2 out]
        n463 = local write "X Axis"(w1017) -> ()
        n464 = local write "Y Axis"(w1017) -> ()
        n465 = local write "Z Axis"(w1017) -> ()
      }
      frame "MagnetometerCal: Update" {
        n466 = Unbundle By Name(w1042) -> ("MagMax"=w1046:dbl[], "MagMin"=w1045:dbl[], "Data"=w1040:dbl[][])
        n467 = Index Array(array=w1040, index (row)=0 ("disabled index (col)")) -> (element=w1038:dbl[])  [unwired: 1 in]
        n468 = for {
          tunnel: w1038 -> [w1048] mode=indexing
          tunnel: w1046 -> [w1049] mode=indexing
          tunnel: w1045 -> [w1047] mode=indexing
          tunnel: [w1052] -> w1044 mode=indexing
          tunnel: [w1051] -> w1043 mode=indexing
          i -> [w1050]
          n469 = Max & Min(x=w1049, y=w1048) -> (max(x,y)=w1052:dbl)  [unwired: 1 out]
          n470 = Max & Min(x=w1047, y=w1048) -> (min(x,y)=w1051:dbl)  [unwired: 1 out]
          n471 = case shown="2" w1050 {
            tunnel: w1047 -> [_ w1056 w1060 w1063]
            tunnel: w1049 -> [_ w1055 w1059 w1064]
            tunnel: w1048 -> [_ w1054 w1058 w1062]
            frame Default {
            }
            frame 0 {
              n472 = Bundle(w1055, w1056, w1054) -> (→"X Axis":cluster{dbl, dbl, dbl})  [unwired: 1 in]
            }
            frame 1 {
              n473 = Bundle(w1059, w1060, w1058) -> (→"Y Axis":cluster{dbl, dbl, dbl})  [unwired: 1 in]
            }
            frame 2 {
              n474 = Bundle(w1064, w1063, w1062) -> (→"Z Axis":cluster{dbl, dbl, dbl})  [unwired: 1 in]
            }
          }
        }
        n475 = Bundle By Name(cluster=w1042, "MagMax"=w1044, "MagMin"=w1043) -> (w1041:T1)
      }
      frame "MagnetometerCal: Generate Cal" {
        n476 = Unbundle By Name(w1082) -> ("MagMax"=w1075:dbl[], "MagMin"=w1074:dbl[])
        n477 = call "NextGUIState.vi"("GUI State"="Clear Queue" ("State"), "Queue In"=w1085) -> ("Queue Out"=w1084:refnum<queue>)  [unwired: 8 in, 1 out]
        n478 = call "NextGUIState.vi"("GUI State"="Clear Serial Comm" ("State"), "Queue In"=w1084) -> ("Queue Out"=w1083:refnum<queue>)  [unwired: 8 in, 1 out]
        n479 = call "LookupCommands.vi"("CommandName"="MagCal") -> ("CommandValue"=w1071:string)  [unwired: 10 in]
        n480 = call "LookupCommands.vi"("CommandName"="MagCalResponse") -> ("CommandValue"=w1065:string)  [unwired: 10 in]
        n481 = for {
          tunnel: w1074 -> [w1107] mode=indexing
          tunnel: w1075 -> [w1103] mode=indexing
          tunnel: [w1102] -> w1078 mode=indexing
          n482 = Compound Arithmetic op=ADD(w1103, invert w1107) -> (w1106:dbl)
          n483 = Divide(x=w1106, y=2.0) -> (x/y=w1104:dbl)
          n484 = Compound Arithmetic op=ADD(w1104, invert w1103) -> (w1102:dbl)
        }
        n485 = Number To Fractional String(number=w1078, precision (6)=i16 6) -> (F-format string=w1095:string[])  [unwired: 2 out]
        n486 = Array To Spreadsheet String(delimiter (Tab)=";", array=w1095, 3:"%s" ("format string")) -> (spreadsheet string=w1098:string)
        n487 = Match Pattern(string=w1098, regular expression="\r\n") -> (before substring=w1091:string)  [unwired: 4 out]
        n488 = Concatenate Strings(w1071, w1091, ";" ("string")) -> (w1066:string)
        n489 = Concatenate Strings(w1066, w1065) -> (w1067:string)
        n490 = call "NextGUIState.vi"("State Argument"=w1067, "GUI State"="Send Command" ("State"), "Queue In"=w1083) -> ("Queue Out"=w1080:refnum<queue>)  [unwired: 7 in, 1 out]
        n491 = call "NextGUIState.vi"("GUI State"="Delay SubPanel", "Queue In"=w1080) -> ("Queue Out"=w1081:refnum<queue>)  [unwired: 8 in, 1 out]
        n492 = Search and Replace String(replace all?=TRUE ("replace all? (F)"), input string=w1091, search string=";", replace string="," ("replace string (\"\")")) -> (result string=w1087:string)  [unwired: 4 in, 3 out]
        n493 = call "NextGUIState.vi"("State Argument"=w1087, "GUI State"="Verify Upload" ("State"), "Queue In"=w1081) -> ("Queue Out"=w1069:refnum<queue>)  [unwired: 7 in, 1 out]
        n494 = call "NextGUIState.vi"("State Argument"=w1066, "GUI State"="Store Calibration", "Queue In"=w1069) -> ("Queue Out"=w1068:refnum<queue>)  [unwired: 7 in, 1 out]
        n495 = call "NextState.vi"("Data"="Calibration Complete" ("State"), "State"="Instructions: Update", "Queue In"=w1068) -> ()  [unwired: 7 in, 2 out]
      }
    }
  }
  n496 = while {
    tunnel: w1 -> [w1109]
    stop <- w1108 stop-if-true
    n497 = event shown="[6] \"ESCCal\": Value Change" {
      selector: _ -> [_ _ _ _ _ _ _ _ _]
      dyn-events: _ -> [_ _ _ _ _ _ _ _ _]
      timeout: _ -> [_ _ _ _ _ _ _ _ _]
      tunnel: w1109 -> [w1112 w1115 w1118 w1120 w1123 w1131 w1140 w1145 w1148]
      tunnel: [FALSE _ _ _ _ _ _ _ _] -> w1108
      event "Upload Flight Software": Value Change {
        n498 = event-data() -> ()  [unwired: 1 in, 1 out]
        n499 = local write "Instruction"("" ("Instruction")) -> ()
        n500 = call "NextStates.vi"("States"=string[] ["TransmitterCal: Hide", "AccelCal: Hide", "MagnetometerCal: Hide", "LargeInstructions: Show", "Response: Disable", "Upload Flight Software"], "Queue In"=w1112) -> ()  [unwired: 8 in, 2 out]
      }
      event "Initialize EEPROM": Value Change {
        n501 = event-data() -> ()  [unwired: 1 in, 1 out]
        n502 = call "NextStates.vi"("States"=string[] ["TransmitterCal: Hide", "AccelCal: Hide", "MagnetometerCal: Hide", "LargeInstructions: Show", "Response: Disable", "EEPROM: Start Initialization"], "Queue In"=w1115) -> ()  [unwired: 8 in, 2 out]
        n503 = local write "Instruction"("" ("Instruction")) -> ()
      }
      event "GyroCal": Value Change {
        n504 = event-data() -> ()  [unwired: 1 in, 1 out]
        n505 = call "NextStates.vi"("States"=string[] ["TransmitterCal: Hide", "AccelCal: Hide", "MagnetometerCal: Hide", "LargeInstructions: Show", "Response: Disable", "GyroCal: Start Cal"], "Queue In"=w1118) -> ()  [unwired: 8 in, 2 out]
        n506 = local write "Instruction"("" ("Instruction")) -> ()
      }
      event "AccelCal": Value Change {
        n507 = event-data() -> ()  [unwired: 1 in, 1 out]
        n508 = call "NextStates.vi"("States"=string[] ["TransmitterCal: Hide", "LargeInstructions: Hide", "MagnetometerCal: Hide", "AccelCal: Show", "Response: Enable", "AccelCal: Start Cal"], "Queue In"=w1120) -> ()  [unwired: 8 in, 2 out]
        n509 = local write "Instruction"("" ("Instruction")) -> ()
      }
      event "MagCal": Value Change {
        n510 = event-data() -> ()  [unwired: 1 in, 1 out]
        n511 = call "NextStates.vi"("States"=string[] ["TransmitterCal: Hide", "LargeInstructions: Hide", "AccelCal: Hide", "MagnetometerCal: Show", "MagnetometerCal: Start Cal"], "Queue In"=w1123) -> ()  [unwired: 8 in, 2 out]
        n512 = local write "Instruction"("" ("Instruction")) -> ()
      }
      event "TransmitterCal": Value Change {
        n513 = event-data() -> ()  [unwired: 1 in, 1 out]
        n514 = call "NextStates.vi"("States"=string[] ["LargeInstructions: Hide", "AccelCal: Hide", "MagnetometerCal: Hide", "TransmitterCal: Show"], "Queue In"=w1131) -> ("Queue Out"=w1127:refnum<queue>)  [unwired: 8 in, 1 out]
        n515 = call "NextGUIState.vi"("GUI State"="Clear Queue", "Queue In"=w1127) -> ("Queue Out"=w1128:refnum<queue>)  [unwired: 8 in, 1 out]
        n516 = call "NextGUIState.vi"("GUI State"="Clear Serial Comm", "Queue In"=w1128) -> ("Queue Out"=w1129:refnum<queue>)  [unwired: 8 in, 1 out]
        n517 = call "NextState.vi"("State"="TransmitterCal: Update Channels", "Queue In"=w1129) -> ()  [unwired: 8 in, 2 out]
      }
      event "ESCCal": Value Change {
        n518 = event-data() -> ()  [unwired: 1 in, 1 out]
        n519 = call "NextStates.vi"("States"=string[] ["TransmitterCal: Hide", "MagnetometerCal: Hide", "AccelCal: Hide", "LargeInstructions: Show", "Response: Disable"], "Queue In"=w1140) -> ("Queue Out"=w1139:refnum<queue>)  [unwired: 8 in, 1 out]
        n520 = call "NextState.vi"("State"="ESCCal: Start Cal", "Queue In"=w1139) -> ("Queue Out"=w1136:refnum<queue>)  [unwired: 8 in, 1 out]
        n521 = call "NextGUIState.vi"("GUI State"="Clear Queue", "Queue In"=w1136) -> ("Queue Out"=w1134:refnum<queue>)  [unwired: 8 in, 1 out]
        n522 = call "NextGUIState.vi"("GUI State"="Clear Serial Comm", "Queue In"=w1134) -> ()  [unwired: 8 in, 2 out]
        n523 = local write "Instruction"("" ("Instruction")) -> ()
      }
      event "OK": Value Change {
        n524 = event-data() -> ()  [unwired: 1 in, 1 out]
        n525 = call "PriorityState.vi"("Data"=enum16{"Wait", "OK", "Cancel"}."OK" ("Reponse"), "State"="Response", "Queue In"=w1145) -> ()  [unwired: 7 in, 2 out]
      }
      event "Cancel": Value Change {
        n526 = event-data() -> ()  [unwired: 1 in, 1 out]
        n527 = call "PriorityState.vi"("Data"=enum16{"Wait", "OK", "Cancel"}."Cancel" ("Reponse"), "State"="Response", "Queue In"=w1148) -> ()  [unwired: 7 in, 2 out]
      }
    }
  }
